vi "DARPA_DoubleJ_20220811_Arduino_ver.vi"() -> ()   [LabVIEW 2021]
uses:
  <vilib>/Instr/_visa.llb/VISA Configure Serial Port (Instr).vi
  <vilib>/FPGAPlugInAG/PCIe-7857/niLvFpga_Open_PCIe-7857.vi
  <vilib>/rvi/interface/common/dynamic/niFpgaDynamicAddResources.vi
  <vilib>/Utility/error.llb/Error Cluster From Error Code.vi
  <vilib>/rvi/errors/niLvFpgaAdjustHostInterfaceError.vi
  <vilib>/FPGAPlugInAG/Dynamic/niLvFpga_Close_Dynamic.vi
  <vilib>/rvi/interface/nirviOpenFPGA/nirviOpenFPGA.xnode
  FPGA Bitfiles/darpatransitionj_FPGATarget_DARPAFPGADoubleJ_E+A750Kw4Ow.lvbitx
  DARPA_FPGA_DoubleJ_20220715.vi
  <vilib>/rvi/interface/nirviReadWriteControl/nirviReadWriteControl.xnode
  <vilib>/rvi/interface/nirviCloseFPGA/nirviCloseFPGA.xnode
  NiFpgaLv.dll
  <vilib>/rvi/interface/Simulation/niFpgaSimulationCallBeginRW.vi
panel:
  out "error out":errorcluster
  in  "stop":bool
  out "Image":u16[][](graph)
  in  "Display":bool=TRUE
  out "Total Frames":i32
  out "Elapsed Time":u32
  out "Software FPS":dbl
  out "Camera FPS":dbl
  in  "H Offset":i32 min=0 max=1604 step=4
  in  "H Width":i32 min=4 max=2304 step=4
  out "SMD":dbl
  out "SHO":i32
  in  "V Offset":i32 min=0 max=1604 step=4
  in  "V Width":i32 min=4 max=2304 step=4
  in  "Binning":u16(ring)=1 items=["1x1"=1, "2x2"=2, "4x4"=4]
  out "SHW":i32
  out "SVO":i32
  out "SVW":i32
  in  "Scan Mode":dbl min=1.0 max=3.0 step=1.0
  in  "Exposure":dbl min=6.576470588235294e-05 max=10.000017235294118 step=1e-08
  out "EXP":dbl
  out "Camera Model":string
  out "Camera Version":string
  out "Camera Serial":string
  in  "Merger on":bool
  in  "ratiocontrol":dbl=1.0
  in  "Arduino COM port":refnum<visa-resource-name>="COM10"
  in  "Arduino \nshut down":bool=TRUE
  in  "Initializer":bool
  out "Serial debugger":string
  in  "PMT2 senstivity":bool
  in  "PMT1 senstivity":bool
  in  "Func amp":bool
  in  "Func Freq":bool
  in  "Func On time":bool
  in  "Func Delay":bool
  in  "PMT1 senstivity input":dbl=0.7 caption="0.5-0.75 V"
  in  "PMT2 senstivity input":dbl caption="0.5-0.75 V"
  in  "Func amp input":dbl=5.0 caption="0 - 5 V"
  in  "Func freq input":dbl=10000.0 caption="100 - 10k Hz"
  in  "Func on Time input":dbl=0.04 caption="0.01 - 1 s"
  in  "Func delay input":dbl caption="0.01 - 1 s"
  out "PMT2 sum":u64(graph)
  out "PMT1 sum":u64(graph)
  out "Unfiltered Signal 1":i16(graph)=643
  out "Filtered Signal 2":i16(graph)=-141
  out "Unfiltered Signal 2":i16(graph)=-138
  in  "Threshold1":dbl=9000.0
  in  "Threshold2":dbl
  out "LabView Timer (sec)":dbl
  out "sample diff":u64
  out "t1 (sample)":u64
  out "t0 (sample)":u64
  out "PMT1 sum":u64
  out "PMT2 sum":u64
  out "Droplet lock on":bool
  out "Filtered Signal1":dbl=373.0
  out "Filtered Signal2":dbl=-141.0
  out "Droplet counter":u64
  out "Unfiltered Signal1":dbl=643.0
  out "Unfiltered Signal2":dbl=-138.0
  in  "Droplet width [ms]":dbl
  in  "determine ratio (xx.xx)":dbl
  out "FPGA loop counter":u64=4737476
  out "Sorted droplet counter":u64
  out "Sort":bool
  in  "FPGA initializer":bool=TRUE
  out "FPGA timer (sec)":dbl=4.737476
  out "FPGA freq":dbl=1000000.0
  out "LabView freq":dbl=8547.008547008547
  out "Filtered Signal 1":i16(graph)=373
  out "PMT1/PMT2":dbl
  out "PMT1/PMT2 (graph)":dbl(graph)
  in  "Shut down program":bool=TRUE
  in  "Set rate1":dbl=1000.0 format="%#_4g"
  in  "Units1":string(combo)="uh"
  in  "Target Vol1":dbl=1000.0 caption="Target Vol (ul)"
  in  "Direction1":string(combo)="inf"
  in  "Send1":bool
  out "Max rate1":dbl=53066.71422466229 format="%#_4g"
  out "Min rate1":dbl=0.7293489203037584 caption="Min rate" format="%#_4g"
  in  "Pump1\nStart/Stop":bool
  out "Dispensed1":string
  in  "Reset1":bool
  out "Remains1":string="1.000000ML"
  in  "Syringe Selection1":string(combo)="BDP1MM"
  in  "dia1 (mm)":dbl=0.1 caption="Set Diameter (mm)" min=0.1 max=50.0
  out "Diameter1 (mm)":dbl=4.699
  in  "Set rate2":dbl=1500.0 format="%#_4g"
  in  "Units2":string(combo)="uh"
  in  "Target Vol2":dbl=2000.0 caption="Target Vol (ul)"
  in  "Direction2":string(combo)="inf"
  out "Max rate2":dbl=54911.979673505 format="%#_4g"
  out "Min rate2":dbl=0.7547102486326527 caption="Min rate" format="%#_4g"
  in  "Syringe Selection2":string(combo)="BDP1MM"
  in  "dia2 (mm)":dbl=0.1 caption="Set Diameter (mm)" min=0.1 max=50.0
  out "Diameter2 (mm)":dbl=4.78
  in  "Set rate3":dbl=1000.0 format="%#_4g"
  in  "Units3":string(combo)="uh"
  in  "Target Vol3":dbl=2000.0 caption="Target Vol (ul)"
  in  "Direction3":string(combo)="inf"
  out "Max rate3":dbl=54911.979673505 format="%#_4g"
  out "Min rate3":dbl=0.7547102486326527 caption="Min rate" format="%#_4g"
  in  "Syringe Selection3":string(combo)="BDP1MM"
  in  "dia3 (mm)":dbl=0.1 caption="Set Diameter (mm)" min=0.1 max=50.0
  out "Diameter3 (mm)":dbl=4.78
  in  "Pump2\nStart/Stop":bool
  in  "Pump3\nStart/Stop":bool
  out "Dispensed2":string
  out "Dispensed3":string
  out "Remains2":string="2.000000ML"
  out "Remains3":string="2.000000ML"
  in  "Reset2":bool
  in  "Reset3":bool
  in  "Reset4":bool
  in  "Syringe COM port":refnum<visa-resource-name>="COM11"
  out "Baud Rate":string="19200"
  in  "Output file path":string="D:\\PhD\\00TAMU\\1.research\\nanoBioSystem\\1.projects\\1.DARPA_iSENTRY\\2.src\\LabView\\transition\\FPGA7857_2020\\output files"
  in  "file name":string="tmep"
  out "Confirm path":string="C:\\Data_JJH\\1.Research\\1.projects\\1.DARPA_iSENTRY\\2.src\\LabView\\transition\\FPGA7857_2020\\output files\\20220811 sorting empty 1to500 1.xls"
  out "Data File Ptr":refnum<file>
  # "For inner peace of developers"
  # "Communication Setting"
  # "Sorting Status"
  # "[Pump1] Syringe Setting"
  # "Arduino setting"
  # "[Pump2] Syringe Setting"
  # "PMT display"
  # "Cockpit"
  # "[Pump3] Syringe Setting"
  # "File saving option"
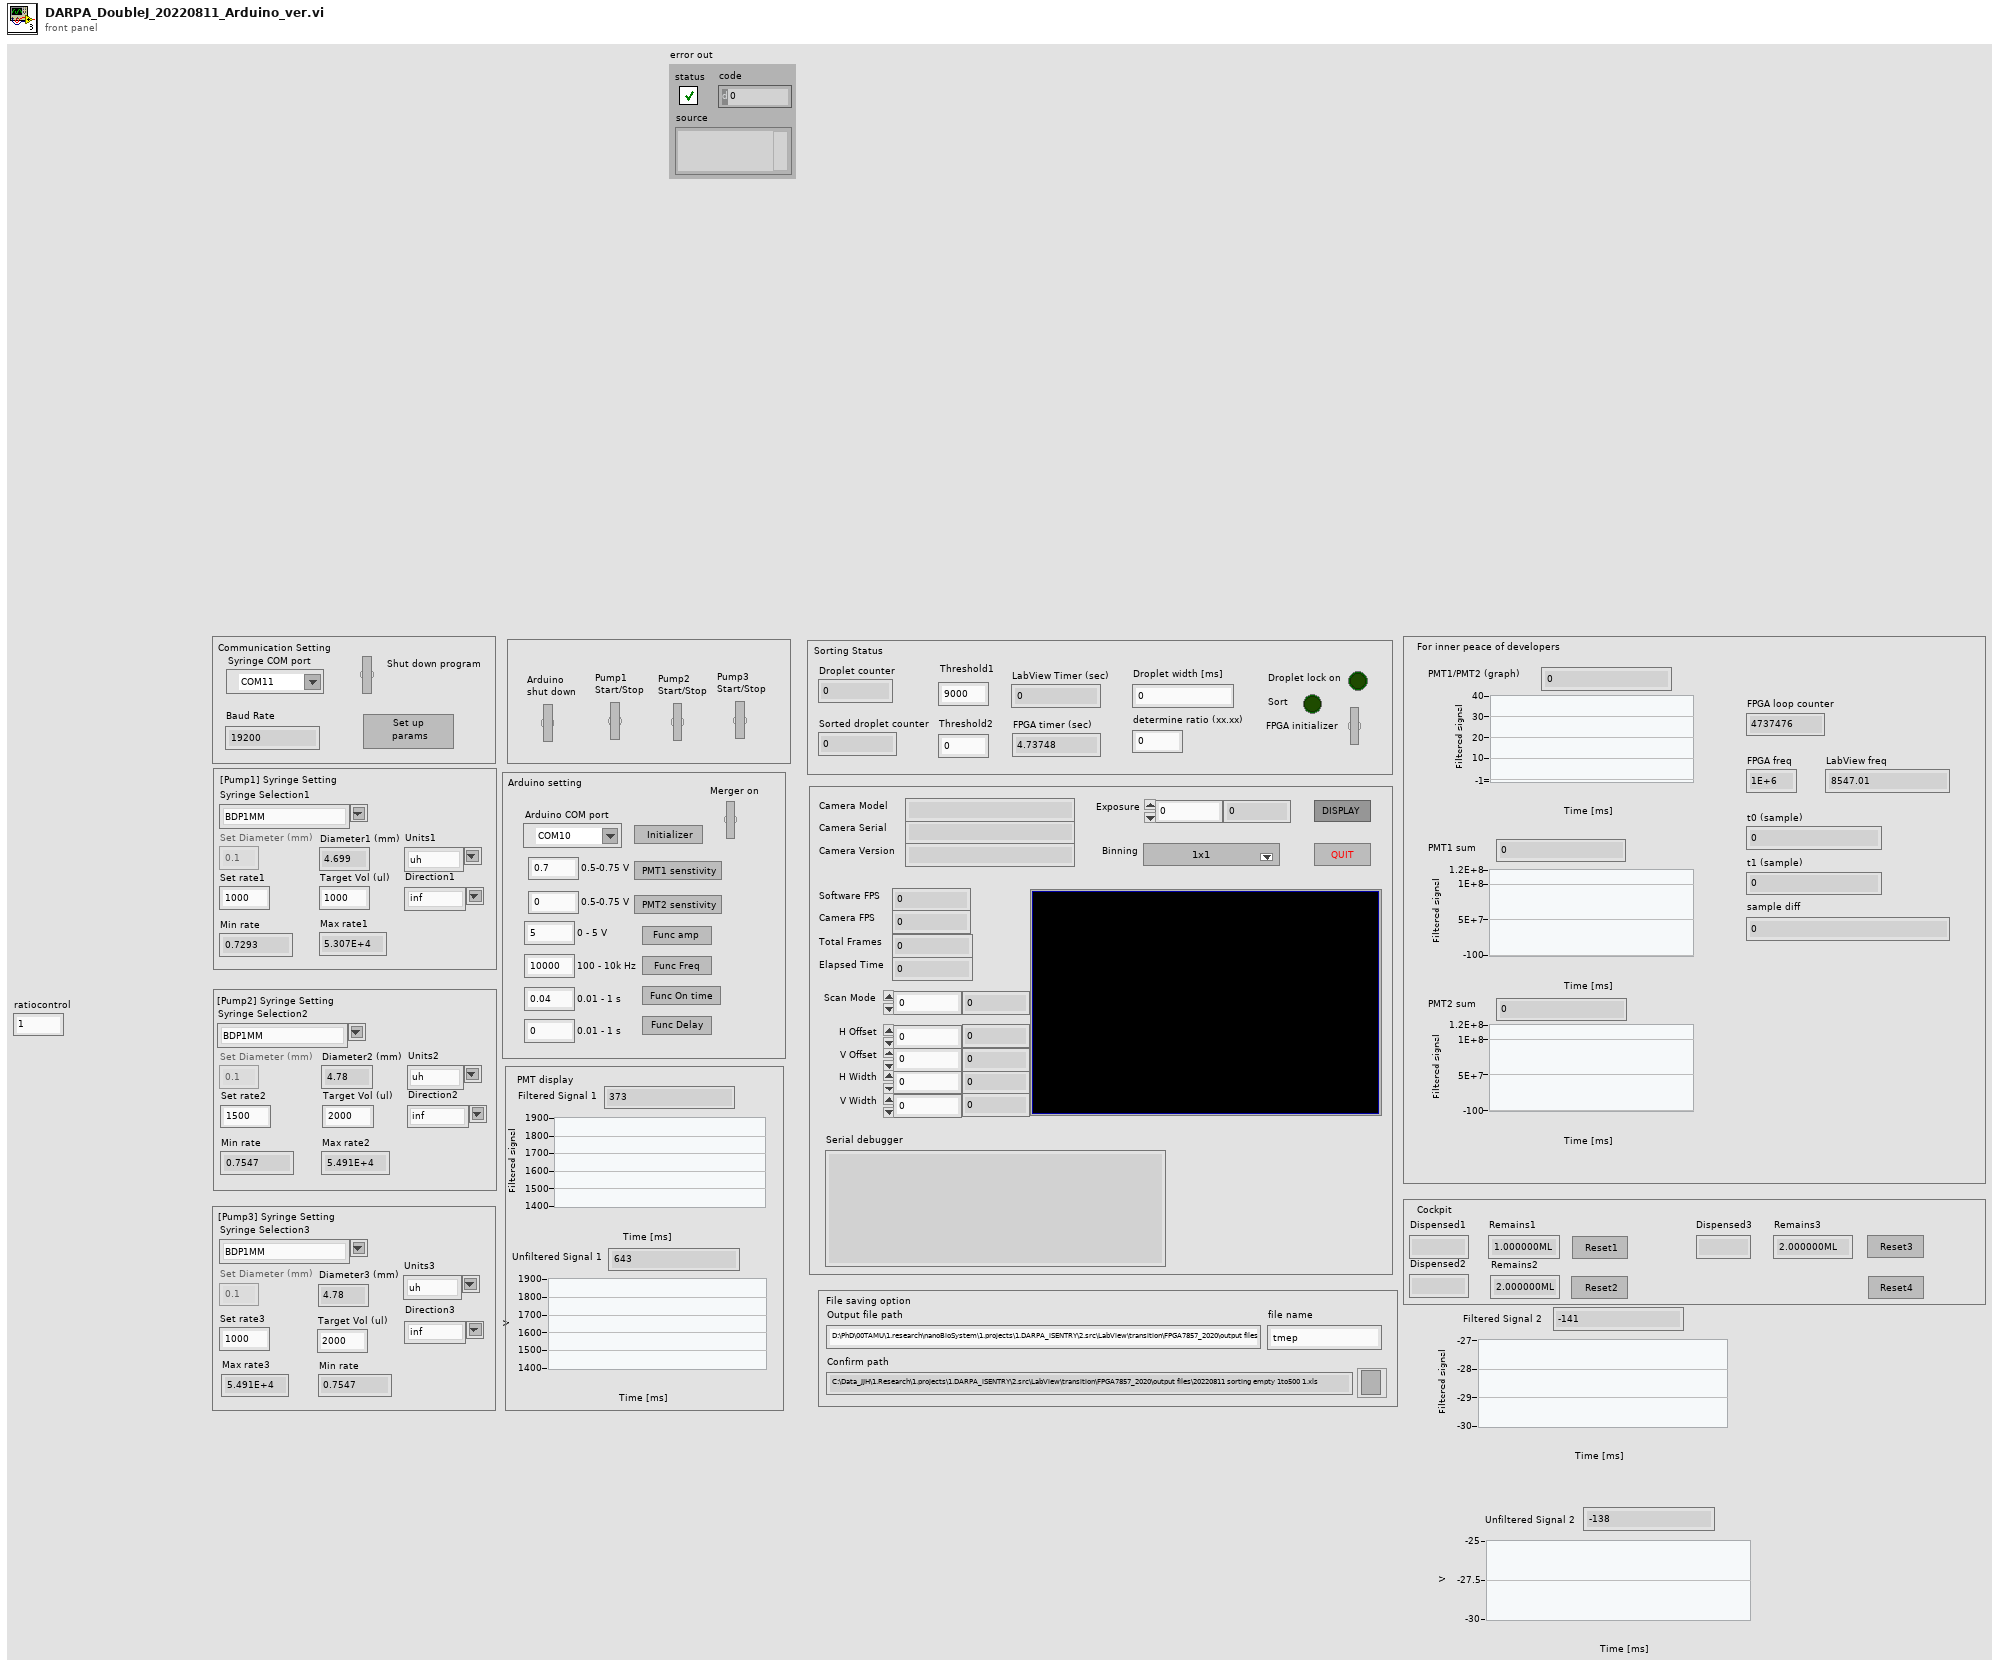
[diagram p1: front panel]
types:
  T1 = enum16{"open", "replace", "create", "open or create", "replace or create", "replace or create with confirmation"}
  T2 = enum8{"Enabled", "Disabled", "Disabled and Grayed Out"}
  T3 = cluster{"Model":string, "Camera ID":string, "Firmware":string}
  T4 = typedef "LVMinMaxIncTypeDef.ctl" = cluster{"Minimum":dbl, "Maximum":dbl, "Increment":dbl}
  T5 = cluster{"H Offset":cluster{"Value":i32, "Limits":T4}, "V Offset":cluster{"Value":i32, "Limits":T4}, "H Size":cluster{"Value":i32, "Limits":T4}, "V Size":cluster{"Value":i32, "Limits":T4}}
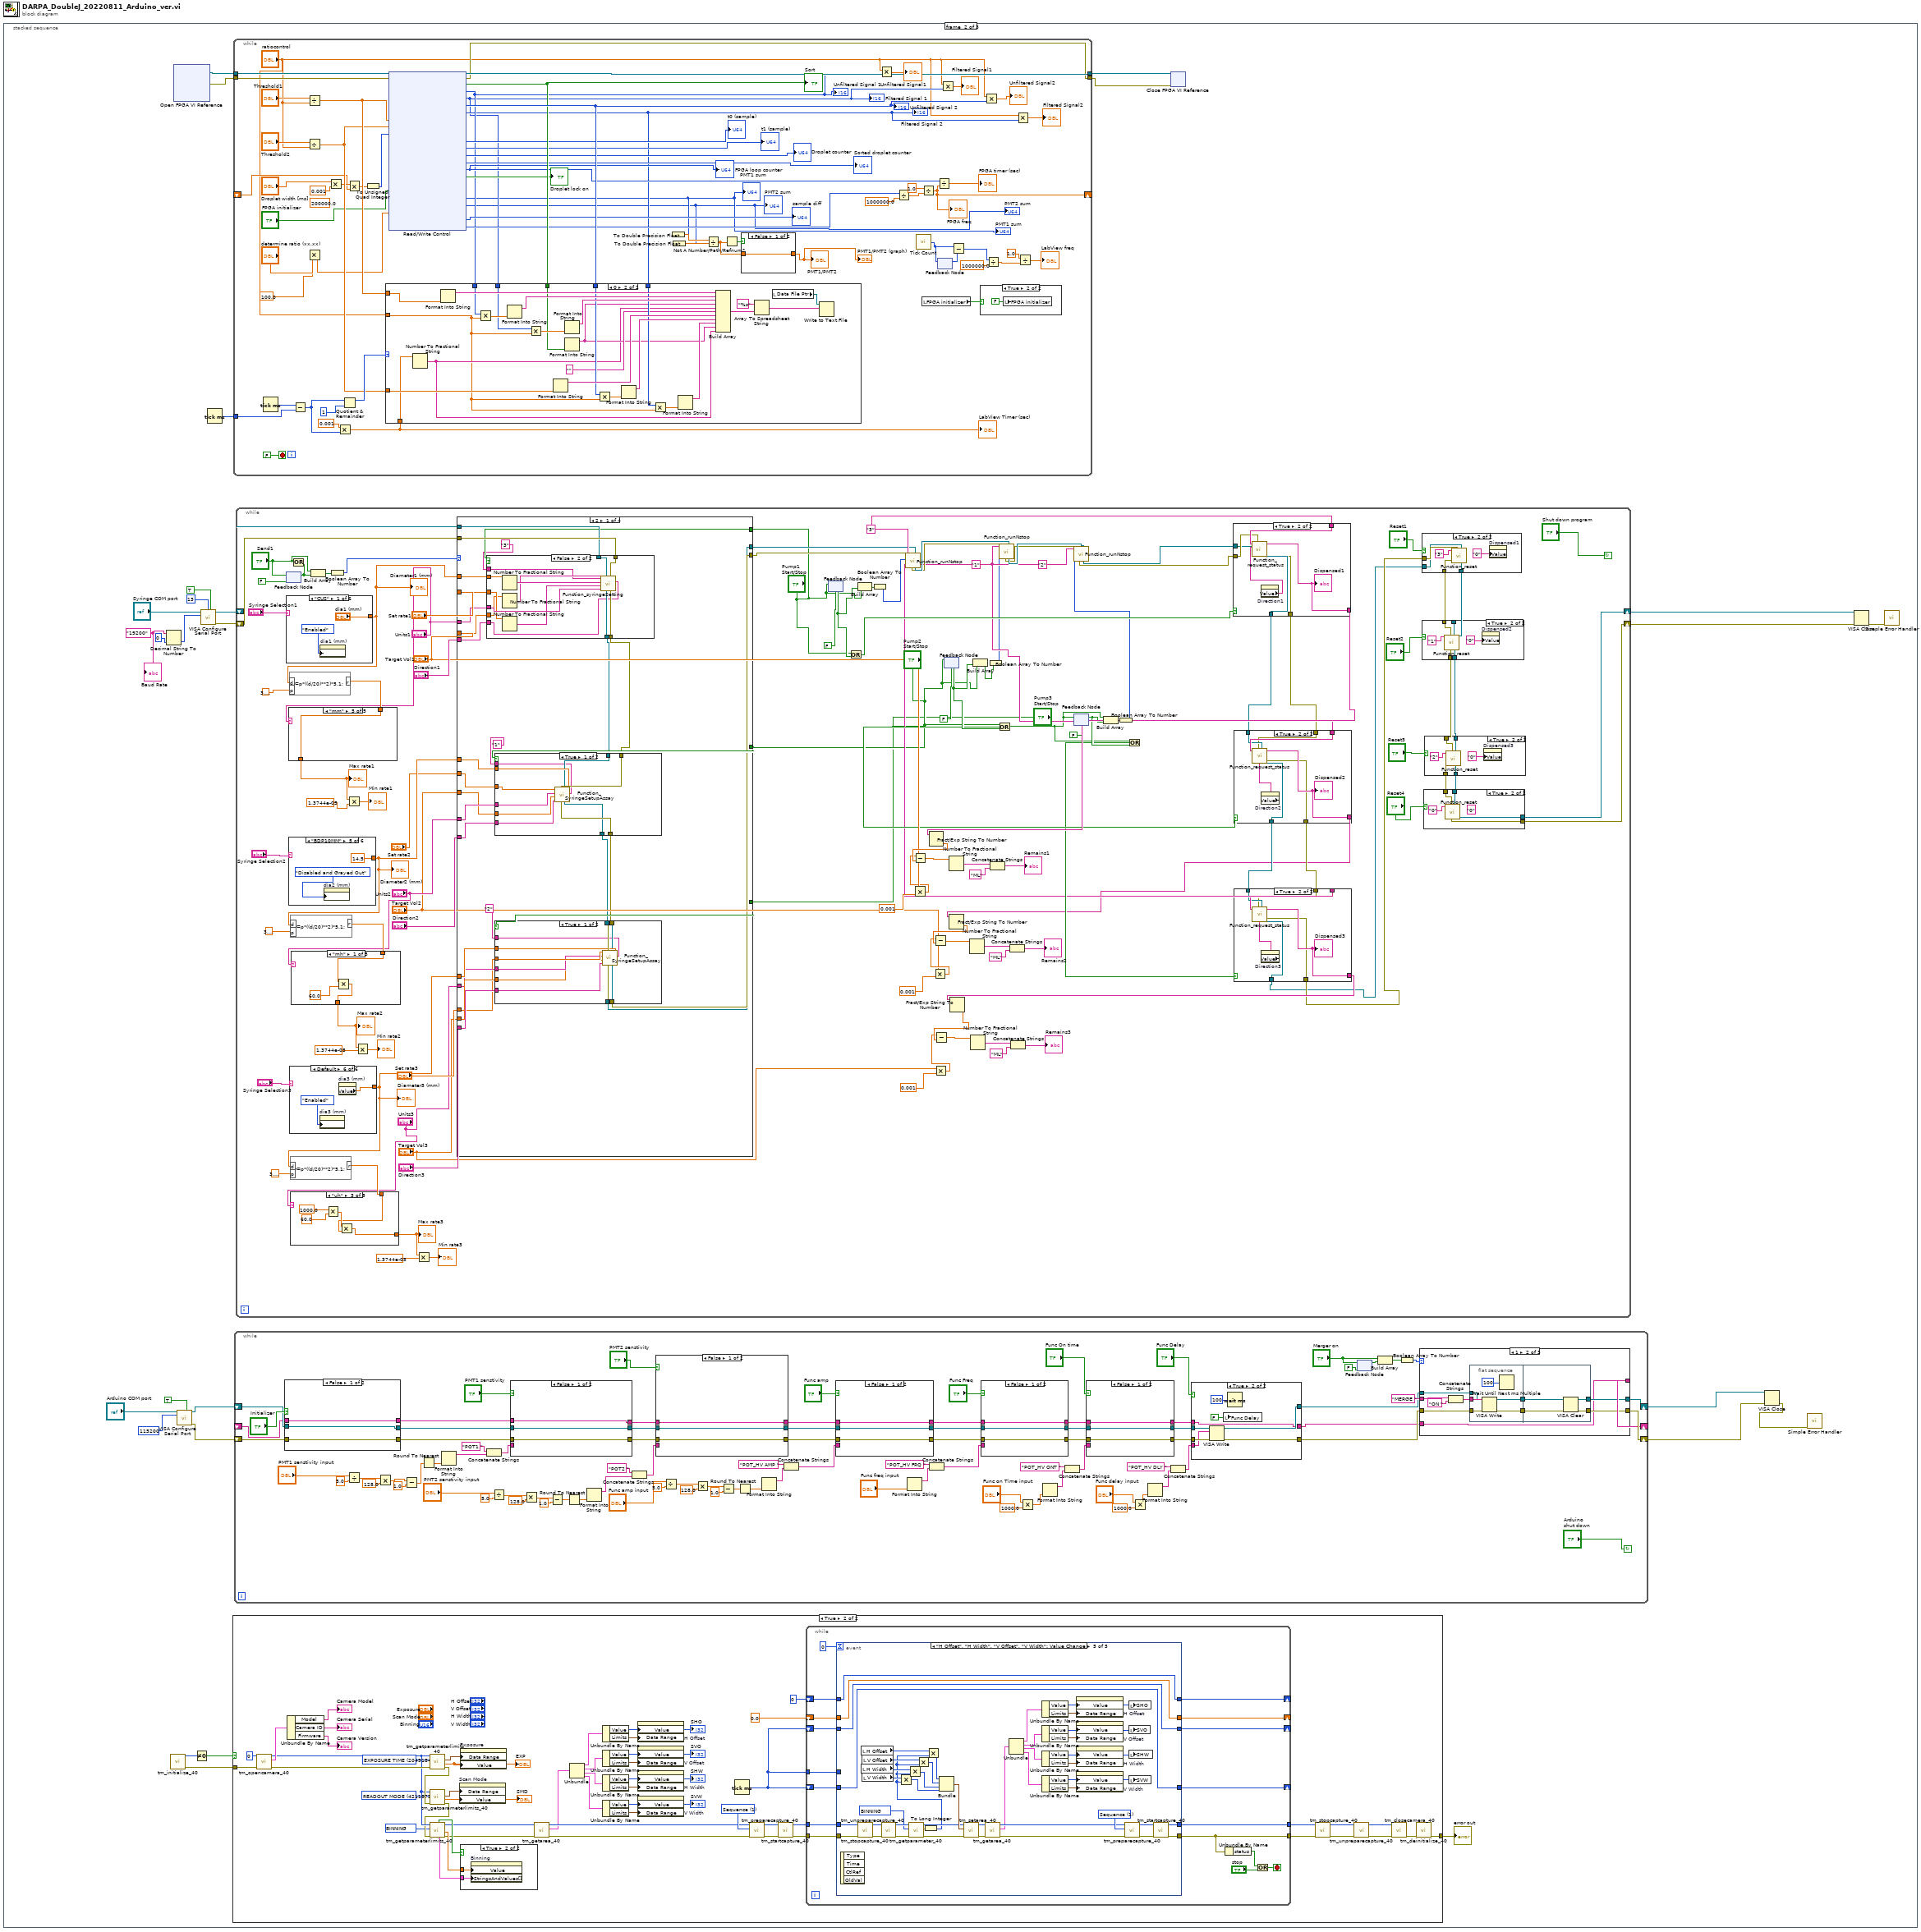
[diagram p0: block diagram]
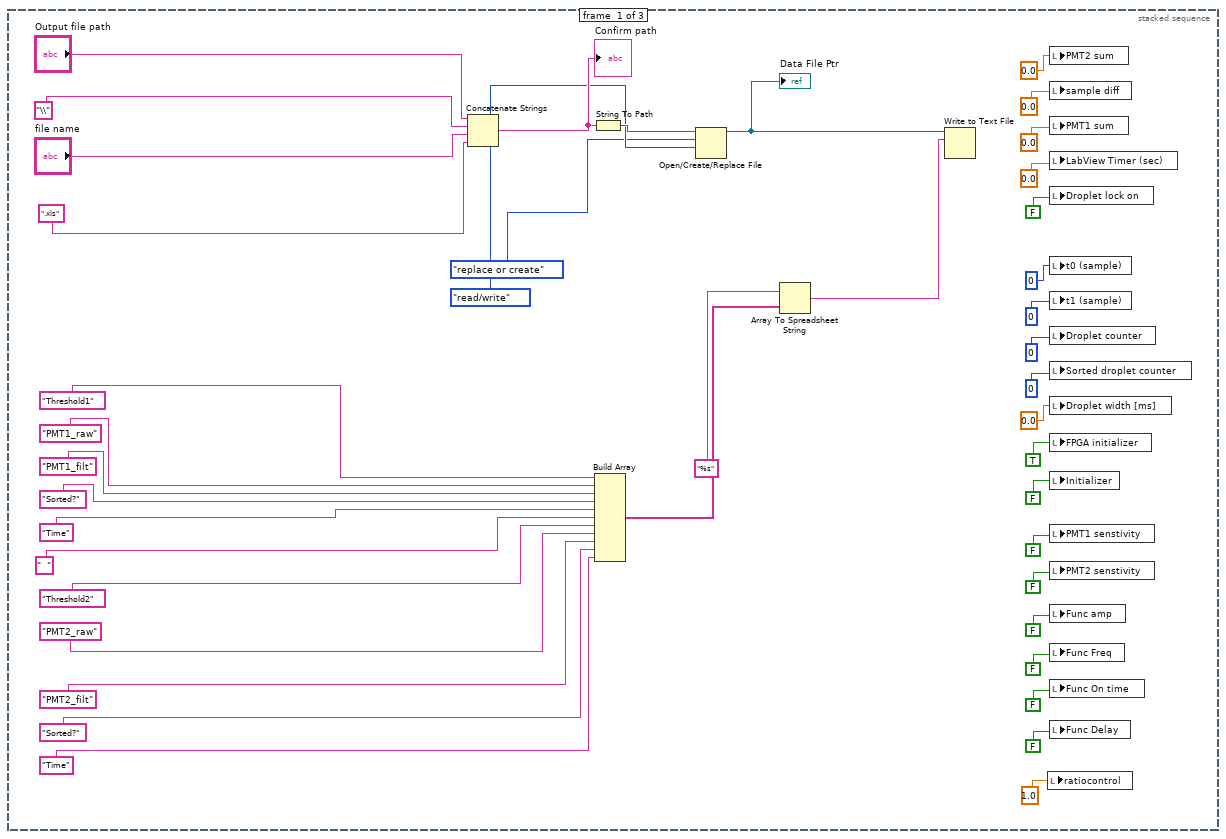
[diagram p2: hidden frame]
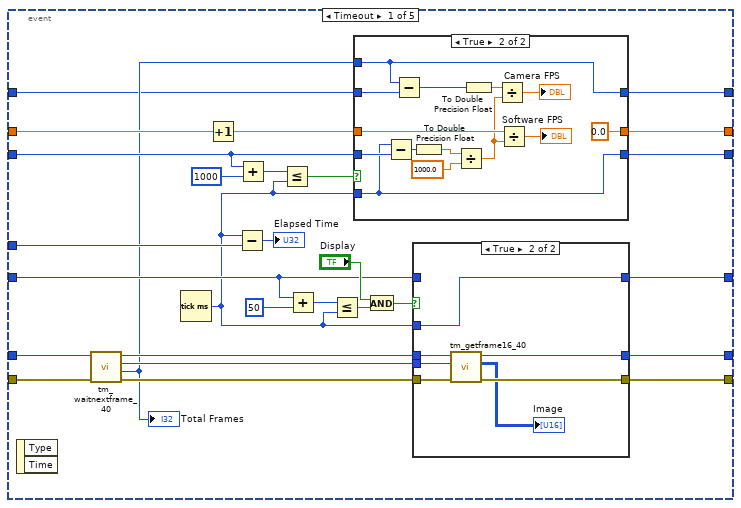
[diagram p5: hidden frame]
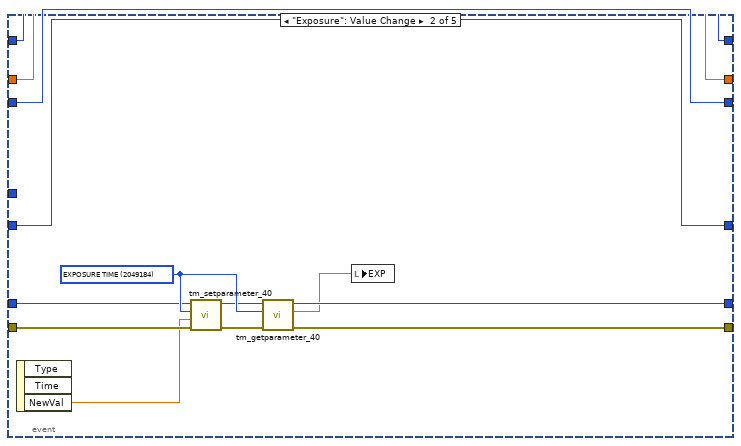
[diagram p8: hidden frame]
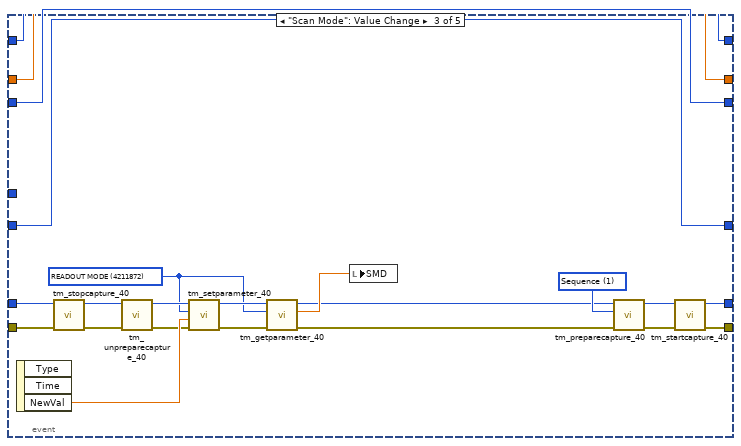
[diagram p9: hidden frame]
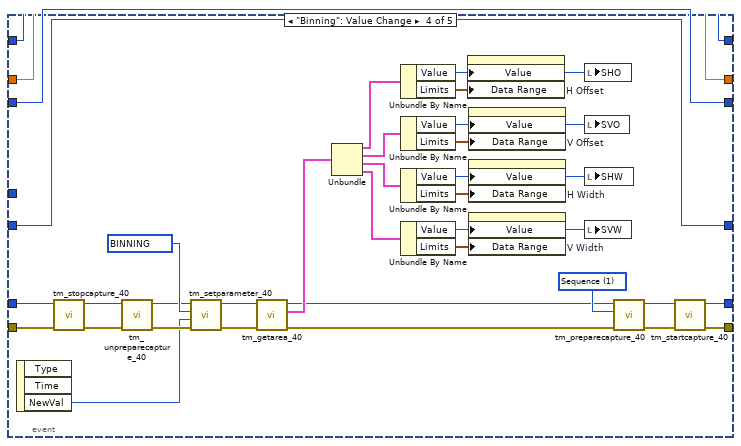
[diagram p10: hidden frame]
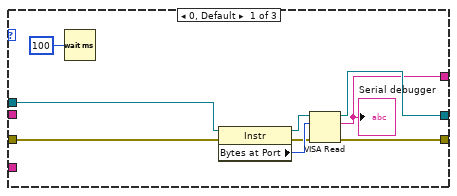
[diagram p11: hidden frame]
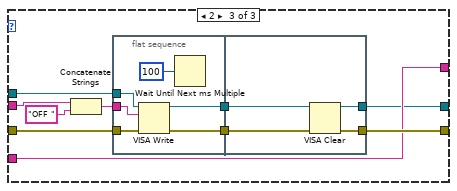
[diagram p12: hidden frame]
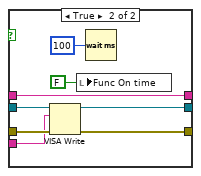
[diagram p14: hidden frame]
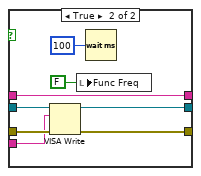
[diagram p15: hidden frame]
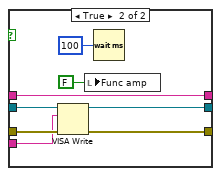
[diagram p16: hidden frame]
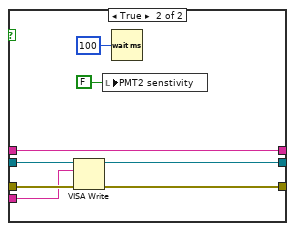
[diagram p17: hidden frame]
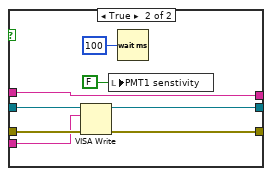
[diagram p18: hidden frame]
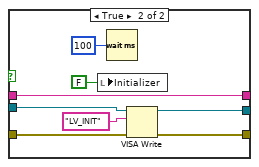
[diagram p19: hidden frame]
diagram:
  n1 = stacked-sequence {
    frame #0 {
      n2 = Concatenate Strings("Output file path", "\\" ("string"), "file name", ".xls" ("string")) -> (w41:string)
      "Confirm path" <- w41
      n3 = String To Path(string=w41) -> (path=w42:path)
      n4 = Build Array("Threshold1", "PMT1_raw", "PMT1_filt", "Sorted?", "Time", "  ", "Threshold2", "PMT2_raw", "PMT2_filt", "Sorted?", "Time") -> (w34:string[])
      n5 = Open/Create/Replace File(file path (use dialog)=w42, operation (0:open)=T1."replace or create", access (0:read/write)=enum16{"read/write", "read-only", "write-only"}."read/write") -> (refnum out=w20:refnum<file>)  [unwired: 3 in, 2 out]
      "Data File Ptr" <- w20
      n6 = Array To Spreadsheet String(array=w34, 3:"%s") -> (spreadsheet string=w22:string)  [unwired: 1 in]
      n7 = Write to Text File(file (use dialog)=w20, text=w22) -> ()  [unwired: 2 in, 3 out]
      n8 = local write "ratiocontrol"(1.0 ("ratiocontrol")) -> ()
      n9 = local write "PMT2 sum"(0.0 ("now")) -> ()
      n10 = local write "sample diff"(0.0 ("sample diff")) -> ()
      n11 = local write "PMT1 sum"(0.0 ("PMT1 sum")) -> ()
      n12 = local write "LabView Timer (sec)"(0.0 ("PMT2 sum")) -> ()
      n13 = local write "Droplet lock on"(FALSE ("Droplet lock on")) -> ()
      n14 = local write "t0 (sample)"(u64 0 ("t0 (sample)")) -> ()
      n15 = local write "t1 (sample)"(u64 0 ("t1 (sample)")) -> ()
      n16 = local write "Droplet counter"(u64 0 ("Droplet counter")) -> ()
      n17 = local write "Sorted droplet counter"(u64 0 ("Sorted droplet counter")) -> ()
      n18 = local write "Droplet width [ms]"(0.0 ("Time compensation [ms]")) -> ()
      n19 = local write "FPGA initializer"(TRUE ("FPGA initializer")) -> ()
      n20 = local write "Initializer"(FALSE ("FPGA initializer")) -> ()
      n21 = local write "PMT1 senstivity"(FALSE ("FPGA initializer")) -> ()
      n22 = local write "PMT2 senstivity"(FALSE ("FPGA initializer")) -> ()
      n23 = local write "Func amp"(FALSE ("FPGA initializer")) -> ()
      n24 = local write "Func Freq"(FALSE ("FPGA initializer")) -> ()
      n25 = local write "Func On time"(FALSE ("FPGA initializer")) -> ()
      n26 = local write "Func Delay"(FALSE ("FPGA initializer")) -> ()
    }
    frame #1 {
      w60 = "19200" ("Baud Rate")
      n27 = Decimal String To Number(string=w60, default (0L)=u32 0 ("default (0 I32)")) -> (number=w63:u32)  [unwired: 1 in, 1 out]
      n28 = call <userlib>:"tm_initialize_40.vi"() -> ("error out"=w44:errorcluster, "Number Of Cameras"=w43:u32)  [unwired: 8 in, 2 out]
      n29 = xnode "Open FPGA VI Reference"() -> ("FPGA VI Reference Out"=w70:refnum<k20>, "error out"=w69:errorcluster)  [unwired: 2 in]
      n30 = call-poly "VISA Configure Serial Port"("VISA resource name"="Arduino COM port", "Enable Termination\nChar (T)"=TRUE ("Enable Termination\nChar (T)"), "baud rate (9600)"=u32 115200) -> ("VISA resource name out"=w50:refnum<visa-resource-name>, "error out"=w49:errorcluster)  [unwired: 11 in]
      n31 = Not Equal To 0?(x=w43) -> (x != 0?=w46:bool)
      n32 = call-poly "VISA Configure Serial Port"("VISA resource name"="Syringe COM port", "termination char\n(0xA = '\\n' = LF)"=u8 13 ("termination char\n(0xA = '\\n' = LF)"), "Enable Termination\nChar (T)"=TRUE ("Enable Termination\nChar (T)"), "baud rate (9600)"=w63) -> ("VISA resource name out"=w59:refnum<visa-resource-name>, "error out"=w58:errorcluster)  [unwired: 10 in]
      n33 = Tick Count (ms)() -> (millisecond timer value=w66:u32)
      n34 = case shown="True" w46 {
        tunnel: [w71 w121] -> w45
        tunnel: w44 -> [w71 w124]
        frame False {
        }
        frame True {
          w93 = u32 2049184 items=["BINNING"=4215968, "BITS PER CHANNEL"=4342976, "ACTIVE VIEW INDEX"=4343136, "CCD MODE"=4212384, "SENSOR MODE"=4212128, "READOUT MODE"=4211872, "EXPOSURE TIME"=2049184, "CONTRAST GAIN"=3163312, "CONTRAST OFFSET"=3163328, "LIGHT MODE"=2114720, "SENSITIVITY"=2114992, "WHITE BALANCE"=3163568, "PHOTON IMAGING MODE"=2115200, "HIGH DYNAMIC RANGE MODE"=3163360, "TRIGGER SOURCE"=1066144, "TRIGGER ACTIVE"=1066160, "TRIGGER MODE"=1066400, "TRIGGER POLARITY"=1066416, "TRIGGER GLOBAL EXPOSURE"=2049680, "FIRST TRIGGER BEHAVIOR"=2049696, "TRIGGER TIMES"=1066448, "OUTPUT TRIGGER POLARITY"=1852592, "OUTPUT TRIGGER DELAY"=1852624, "OUTPUT TRIGGER PERIOD"=1852640, "TEMPERATURE"=2115232, "TEMPERATURE TARGET"=2115264, "SENSOR COOLER FAN"=2115296, "MECHANICAL SHUTTER"=2115488, "BACK FOCUS POSITION"=8422304, "FRAMEBUNDLE MODE"=4346784, "FRAMEBUNDLE NUMBER"=4346800, "LINEBUNDLE HEIGHT"=4212192, "TRIGGER CONNECTOR"=1066432, "IMAGE PIXEL TYPE"=4343296, "OUTPUT TRIGGER KIND"=1852656, "READOUT DIRECTION"=4211904, "CHANNEL SYNC"=1852352] ("Parameter")
          w94 = u32 4211872 items=["BINNING"=4215968, "BITS PER CHANNEL"=4342976, "ACTIVE VIEW INDEX"=4343136, "CCD MODE"=4212384, "SENSOR MODE"=4212128, "READOUT MODE"=4211872, "EXPOSURE TIME"=2049184, "CONTRAST GAIN"=3163312, "CONTRAST OFFSET"=3163328, "LIGHT MODE"=2114720, "SENSITIVITY"=2114992, "WHITE BALANCE"=3163568, "PHOTON IMAGING MODE"=2115200, "HIGH DYNAMIC RANGE MODE"=3163360, "TRIGGER SOURCE"=1066144, "TRIGGER ACTIVE"=1066160, "TRIGGER MODE"=1066400, "TRIGGER POLARITY"=1066416, "TRIGGER GLOBAL EXPOSURE"=2049680, "FIRST TRIGGER BEHAVIOR"=2049696, "TRIGGER TIMES"=1066448, "OUTPUT TRIGGER POLARITY"=1852592, "OUTPUT TRIGGER DELAY"=1852624, "OUTPUT TRIGGER PERIOD"=1852640, "TEMPERATURE"=2115232, "TEMPERATURE TARGET"=2115264, "SENSOR COOLER FAN"=2115296, "MECHANICAL SHUTTER"=2115488, "BACK FOCUS POSITION"=8422304, "FRAMEBUNDLE MODE"=4346784, "FRAMEBUNDLE NUMBER"=4346800, "LINEBUNDLE HEIGHT"=4212192, "TRIGGER CONNECTOR"=1066432, "IMAGE PIXEL TYPE"=4343296, "OUTPUT TRIGGER KIND"=1852656, "READOUT DIRECTION"=4211904, "CHANNEL SYNC"=1852352] ("Parameter")
          w95 = u32 4215968 items=["BINNING"=4215968, "BITS PER CHANNEL"=4342976, "ACTIVE VIEW INDEX"=4343136, "CCD MODE"=4212384, "SENSOR MODE"=4212128, "READOUT MODE"=4211872, "EXPOSURE TIME"=2049184, "CONTRAST GAIN"=3163312, "CONTRAST OFFSET"=3163328, "LIGHT MODE"=2114720, "SENSITIVITY"=2114992, "WHITE BALANCE"=3163568, "PHOTON IMAGING MODE"=2115200, "HIGH DYNAMIC RANGE MODE"=3163360, "TRIGGER SOURCE"=1066144, "TRIGGER ACTIVE"=1066160, "TRIGGER MODE"=1066400, "TRIGGER POLARITY"=1066416, "TRIGGER GLOBAL EXPOSURE"=2049680, "FIRST TRIGGER BEHAVIOR"=2049696, "TRIGGER TIMES"=1066448, "OUTPUT TRIGGER POLARITY"=1852592, "OUTPUT TRIGGER DELAY"=1852624, "OUTPUT TRIGGER PERIOD"=1852640, "TEMPERATURE"=2115232, "TEMPERATURE TARGET"=2115264, "SENSOR COOLER FAN"=2115296, "MECHANICAL SHUTTER"=2115488, "BACK FOCUS POSITION"=8422304, "FRAMEBUNDLE MODE"=4346784, "FRAMEBUNDLE NUMBER"=4346800, "LINEBUNDLE HEIGHT"=4212192, "TRIGGER CONNECTOR"=1066432, "IMAGE PIXEL TYPE"=4343296, "OUTPUT TRIGGER KIND"=1852656, "READOUT DIRECTION"=4211904, "CHANNEL SYNC"=1852352] ("Parameter")
          w119 = 1 items=["Snap", "Sequence"] ("Capture mode")
          n35 = call <userlib>:"tm_opencamera_40.vi"("error in (no error)"=w124, "Camera Index"=u32 0) -> ("error out"=w102:errorcluster, "Camera Details"=w106:T3, "Handle out"=w100:u32)  [unwired: 7 in]
          n36 = Unbundle By Name(w106) -> ("Model"=→"Camera Model":string, "Camera ID"=→"Camera Serial":string, "Firmware"=→"Camera Version":string)
          n37 = call <userlib>:"tm_getparameterlimits_40.vi"("error in (no error)"=w102, "Parameter"=w93, "Handle in"=w100) -> ("error out"=w101:errorcluster, "default"=w85:dbl, "Range"=w86:cluster{"min":dbl, "max":dbl, "step":dbl})  [unwired: 2 in, 4 out]
          "EXP" <- w85
          n38 = call <userlib>:"tm_getparameterlimits_40.vi"("error in (no error)"=w101, "Parameter"=w94, "Handle in"=w100) -> ("error out"=w99:errorcluster, "default"=w87:dbl, "Range"=w88:cluster{"min":dbl, "max":dbl, "step":dbl})  [unwired: 2 in, 4 out]
          "SMD" <- w87
          n39 = call <userlib>:"tm_getparameterlimits_40.vi"("error in (no error)"=w99, "Parameter"=w95, "Handle in"=w100) -> ("error out"=w92:errorcluster, "default"=w97:dbl, "Handle out"=w91:u32, "Value Names"=w96:cluster{"Name":string, "Value":dbl}[], "Writable"=w98:bool)  [unwired: 2 in, 2 out]
          n40 = property on="Scan Mode" class="DigNum (strict)"("Data Range"=w88, "Value"=w87) -> ()  [unwired: 2 in, 2 out]
          n41 = property on="Exposure" class="DigNum (strict)"("Data Range"=w86, "Value"=w85) -> ()  [unwired: 2 in, 2 out]
          n42 = case shown="True" w98 {
            tunnel: w96 -> [_ w126]
            tunnel: w97 -> [_ w125]
            frame False {
            }
            frame True {
              n43 = property on="Binning" class="Ring (strict)"("Value"=w125, "StringsAndValues[]"=w126) -> ()  [unwired: 2 in, 2 out]
            }
          }
          n44 = call <userlib>:"tm_getarea_40.vi"("error in (no error)"=w92, "Handle in"=w91) -> ("error out"=w90:errorcluster, "Sub Region"=w80:T5, "Handle out"=w89:u32)  [unwired: 7 in]
          n45 = Unbundle(w80) -> ("H Offset"=w84:cluster{"Value":i32, "Limits":T4}, "V Offset"=w83:cluster{"Value":i32, "Limits":T4}, "H Size"=w82:cluster{"Value":i32, "Limits":T4}, "V Size"=w81:cluster{"Value":i32, "Limits":T4})
          n46 = Unbundle By Name(w84) -> ("Value"=w79:i32, "Limits"=w78:T4)
          "SHO" <- w79
          n47 = Unbundle By Name(w83) -> ("Value"=w73:i32, "Limits"=w72:T4)
          "SVO" <- w73
          n48 = Unbundle By Name(w82) -> ("Value"=w75:i32, "Limits"=w74:T4)
          "SHW" <- w75
          n49 = Unbundle By Name(w81) -> ("Value"=w77:i32, "Limits"=w76:T4)
          "SVW" <- w77
          n50 = property on="H Offset" class="DigNum (strict)"("Value"=w79, "Data Range"=w78) -> ()  [unwired: 2 in, 2 out]
          n51 = property on="V Offset" class="DigNum (strict)"("Value"=w73, "Data Range"=w72) -> ()  [unwired: 2 in, 2 out]
          n52 = property on="H Width" class="DigNum (strict)"("Value"=w75, "Data Range"=w74) -> ()  [unwired: 2 in, 2 out]
          n53 = property on="V Width" class="DigNum (strict)"("Value"=w77, "Data Range"=w76) -> ()  [unwired: 2 in, 2 out]
          n54 = Tick Count (ms)() -> (millisecond timer value=w114:u32)
          n55 = call <userlib>:"tm_preparecapture_40.vi"("error in (no error)"=w90, "Capture mode"=w119, "Handle in"=w89) -> ("error out"=w117:errorcluster, "Handle out"=w118:u32)  [unwired: 5 in, 2 out]
          n56 = call <userlib>:"tm_startcapture_40.vi"("error in (no error)"=w117, "Handle in"=w118) -> ("error out"=w116:errorcluster, "Handle out"=w115:u32)  [unwired: 8 in]
          n57 = while {
            tunnel: w116 -> [w133]
            tunnel: [w131] -> w113
            tunnel: [w130] -> w112
            shift-right: [w139] -> _
            shift-left: w114 -> [w137]
            shift-right: [w140] -> _
            shift-left: 0.0 -> [w138]
            shift-right: [w132] -> _
            shift-left: w114 -> [w135]
            tunnel: w115 -> [w134]
            tunnel: w114 -> [w136]
            shift-right: [w127] -> _
            shift-left: 0 -> [w128]
            stop <- w141 stop-if-true
            n58 = event shown="[4] \"H Offset\", \"H Width\", \"V Offset\", \"V Width\": Value Change" {
              selector: _ -> [_ _ _ _ _]
              dyn-events: _ -> [_ _ _ _ _]
              timeout: 0 -> [_ _ _ _ _]
              tunnel: [w148 w209 w231 w260 w306] -> w140
              tunnel: [w147 w210 w232 w261 w307] -> w139
              tunnel: w138 -> [w157 w209 w231 w260 w306]
              tunnel: w137 -> [w150 w210 w232 w261 w307]
              tunnel: w136 -> [w153 _ _ _ _]
              tunnel: w135 -> [w158 w211 w233 w267 w313]
              tunnel: w134 -> [w160 w204 w228 w259 w304]
              tunnel: w133 -> [w159 w206 w227 w258 w303]
              tunnel: [w156 w211 w233 w267 w313] -> w132
              tunnel: [w155 w201 w222 w262 w308] -> w131
              tunnel: [w154 w199 w223 w263 w309] -> w130
              tunnel: w128 -> [w145 w208 w221 w255 w300]
              tunnel: [w144 w208 w221 w255 w300] -> w127
              event Timeout {
                n59 = event-data() -> ()  [unwired: 1 in, 2 out]
                n60 = call <userlib>:"tm_waitnextframe_40.vi"("error in (no error)"=w159, "Handle in"=w160) -> ("error out"=w164:errorcluster, "Frame Count"=w146:i32, "Frame Index"=w163:i32, "Handle out"=w165:u32)  [unwired: 6 in]
                "Total Frames" <- w146
                n61 = Tick Count (ms)() -> (millisecond timer value=w152:u32)
                n62 = Increment(x=w157) -> (x+1=w149:dbl)
                n63 = Subtract(x=w152, y=w153) -> (x-y=→"Elapsed Time":u32)
                n64 = Add(x=w150, y=u32 1000) -> (x+y=w171:u32)
                n65 = Less Or Equal?(x=w171, y=w152) -> (x <= y?=w151:bool)
                n66 = Add(x=w158, y=u32 50) -> (x+y=w169:u32)
                n67 = Less Or Equal?(x=w169, y=w152) -> (x <= y?=w167:bool)
                n68 = case shown="True" w151 {
                  tunnel: w150 -> [w174 w183]
                  tunnel: [w174 w180] -> w147
                  tunnel: w149 -> [w173 w186]
                  tunnel: w152 -> [_ w180]
                  tunnel: [w173 0.0] -> w148
                  tunnel: w146 -> [_ w175]
                  tunnel: w145 -> [w172 w178]
                  tunnel: [w172 w175] -> w144
                  frame False {
                  }
                  frame True {
                    n69 = Subtract(x=w180, y=w183) -> (x-y=w182:u32)
                    n70 = Subtract(x=w175, y=w178) -> (x-y=w176:i32)
                    n71 = To Double Precision Float(number=w182) -> (double precision float=w188:dbl)
                    n72 = Divide(x=w188, y=1000.0) -> (x/y=w179:dbl)
                    n73 = To Double Precision Float(number=w176) -> (double precision float=w177:dbl)
                    n74 = Divide(x=w177, y=w179) -> (x/y=→"Camera FPS":dbl)
                    n75 = Divide(x=w186, y=w179) -> (x/y=→"Software FPS":dbl)
                  }
                }
                n76 = And(x="Display", y=w167) -> (x .and. y?=w162:bool)
                n77 = case shown="True" w162 {
                  tunnel: w158 -> [w191 _]
                  tunnel: w152 -> [_ w198]
                  tunnel: [w191 w198] -> w156
                  tunnel: w165 -> [w190 w197]
                  tunnel: w164 -> [w189 w196]
                  tunnel: [w190 w195] -> w155
                  tunnel: [w189 w194] -> w154
                  tunnel: w163 -> [_ w192]
                  frame False {
                  }
                  frame True {
                    n78 = call <userlib>:"tm_getframe16_40.vi"("error in (no error)"=w196, "Frame Index"=w192, "Handle in"=w197) -> ("error out"=w194:errorcluster, "Data"=→"Image":u16[][], "Handle out"=w195:u32)  [unwired: 5 in, 1 out]
                  }
                }
              }
              event "Exposure": Value Change {
                w207 = u32 2049184 items=["SENSOR MODE"=4212128, "CCD MODE"=4212384, "READOUT MODE"=4211872, "ACTIVE VIEW INDEX"=4343136, "BITS PER CHANNEL"=4342976, "IMAGE PIXEL TYPE"=4343296, "BINNING"=4215968, "EXPOSURE TIME"=2049184, "CONTRAST GAIN"=3163312, "CONTRAST OFFSET"=3163328, "LIGHT MODE"=2114720, "SENSITIVITY"=2114992, "PHOTON IMAGING MODE"=2115200, "HIGH DYNAMIC RANGE MODE"=3163360, "WHITE BALANCE"=3163568, "TEMPERATURE"=2115232, "TEMPERATURE TARGET"=2115264, "SENSOR COOLER FAN"=2115296, "LINEBUNDLE HEIGHT"=4212192, "MECHANICAL SHUTTER"=2115488, "BACK FOCUS POSITION"=8422304, "TRIGGER CONNECTOR"=1066432, "TRIGGER SOURCE"=1066144, "OUTPUT TRIGGER SOURCE"=1852576, "TRIGGER GLOBAL EXPOSURE"=2049680, "FIRST TRIGGER BEHAVIOR"=2049696, "CHANNEL SYNC"=1852352, "READOUT DIRECTION"=4211904, "PRE HSYNC COUNT"=1852704] ("Parameter")
                n79 = event-data() -> ("NewVal"=w205:dbl)  [unwired: 1 in, 2 out]
                n80 = call <userlib>:"tm_setparameter_40.vi"("error in (no error)"=w206, "Value in"=w205, "Parameter"=w207, "Handle in"=w204) -> ("error out"=w203:errorcluster, "Handle out"=w202:u32)  [unwired: 6 in]
                n81 = call <userlib>:"tm_getparameter_40.vi"("error in (no error)"=w203, "Parameter"=w207, "Handle in"=w202) -> ("error out"=w199:errorcluster, "Value out"=w200:dbl, "Handle out"=w201:u32)  [unwired: 6 in]
                n82 = local write "EXP"(w200) -> ()
              }
              event "Scan Mode": Value Change {
                w212 = u32 4211872 items=["SENSOR MODE"=4212128, "CCD MODE"=4212384, "READOUT MODE"=4211872, "ACTIVE VIEW INDEX"=4343136, "BITS PER CHANNEL"=4342976, "IMAGE PIXEL TYPE"=4343296, "BINNING"=4215968, "EXPOSURE TIME"=2049184, "CONTRAST GAIN"=3163312, "CONTRAST OFFSET"=3163328, "LIGHT MODE"=2114720, "SENSITIVITY"=2114992, "PHOTON IMAGING MODE"=2115200, "HIGH DYNAMIC RANGE MODE"=3163360, "WHITE BALANCE"=3163568, "TEMPERATURE"=2115232, "TEMPERATURE TARGET"=2115264, "SENSOR COOLER FAN"=2115296, "LINEBUNDLE HEIGHT"=4212192, "MECHANICAL SHUTTER"=2115488, "BACK FOCUS POSITION"=8422304, "TRIGGER CONNECTOR"=1066432, "TRIGGER SOURCE"=1066144, "OUTPUT TRIGGER SOURCE"=1852576, "TRIGGER GLOBAL EXPOSURE"=2049680, "FIRST TRIGGER BEHAVIOR"=2049696, "CHANNEL SYNC"=1852352, "READOUT DIRECTION"=4211904, "PRE HSYNC COUNT"=1852704] ("Parameter")
                w226 = 1 items=["Snap", "Sequence"] ("Capture mode")
                n83 = event-data() -> ("NewVal"=w217:dbl)  [unwired: 1 in, 2 out]
                n84 = call <userlib>:"tm_stopcapture_40.vi"("error in (no error)"=w227, "Handle in"=w228) -> ("error out"=w229:errorcluster, "Handle out"=w230:u32)  [unwired: 8 in]
                n85 = call <userlib>:"tm_unpreparecapture_40.vi"("error in (no error)"=w229, "Handle in"=w230) -> ("error out"=w215:errorcluster, "Handle out"=w216:u32)  [unwired: 8 in]
                n86 = call <userlib>:"tm_setparameter_40.vi"("error in (no error)"=w215, "Value in"=w217, "Parameter"=w212, "Handle in"=w216) -> ("error out"=w214:errorcluster, "Handle out"=w213:u32)  [unwired: 6 in]
                n87 = call <userlib>:"tm_getparameter_40.vi"("error in (no error)"=w214, "Parameter"=w212, "Handle in"=w213) -> ("error out"=w220:errorcluster, "Value out"=w219:dbl, "Handle out"=w218:u32)  [unwired: 6 in]
                n88 = local write "SMD"(w219) -> ()
                n89 = call <userlib>:"tm_preparecapture_40.vi"("error in (no error)"=w220, "Capture mode"=w226, "Handle in"=w218) -> ("error out"=w224:errorcluster, "Handle out"=w225:u32)  [unwired: 5 in, 2 out]
                n90 = call <userlib>:"tm_startcapture_40.vi"("error in (no error)"=w224, "Handle in"=w225) -> ("error out"=w223:errorcluster, "Handle out"=w222:u32)  [unwired: 8 in]
              }
              event "Binning": Value Change {
                w253 = u32 4215968 items=["BINNING"=4215968, "BITS PER CHANNEL"=2, "ACTIVE VIEW INDEX"=3, "CCD MODE"=4, "SENSOR MODE"=5, "READOUT MODE"=6, "EXPOSURE TIME"=7, "CONTRAST GAIN"=8, "CONTRAST OFFSET"=9, "LIGHT MODE"=10, "SENSITIVITY"=11, "WHITE BALANCE"=12, "PHOTON IMAGING MODE"=13, "HIGH DYNAMIC RANGE MODE"=14, "TRIGGER SOURCE"=15, "TRIGGER ACTIVE"=16, "TRIGGER MODE"=17, "TRIGGER POLARITY"=18, "TRIGGER GLOBAL EXPOSURE"=19, "FIRST TRIGGER BEHAVIOR"=20, "TRIGGER TIMES"=21, "OUTPUT TRIGGER POLARITY"=22, "OUTPUT TRIGGER DELAY"=23, "OUTPUT TRIGGER PERIOD"=24, "TEMPERATURE"=25, "TEMPERATURE TARGET"=26, "SENSOR COOLER FAN"=27, "MECHANICAL SHUTTER"=28, "BACK FOCUS POSITION"=29, "FRAMEBUNDLE MODE"=30, "FRAMEBUNDLE NUMBER"=31, "LINEBUNDLE HEIGHT"=32, "TRIGGER CONNECTOR"=33, "IMAGE PIXEL TYPE"=34, "OUTPUT TRIGGER KIND"=35, "READOUT DIRECTION"=36, "CHANNEL SYNC"=37] ("Parameter")
                w266 = 1 items=["Snap", "Sequence"] ("Capture mode")
                n91 = event-data() -> ("NewVal"=w251:u16)  [unwired: 1 in, 2 out]
                n92 = call <userlib>:"tm_stopcapture_40.vi"("error in (no error)"=w258, "Handle in"=w259) -> ("error out"=w256:errorcluster, "Handle out"=w257:u32)  [unwired: 8 in]
                n93 = call <userlib>:"tm_unpreparecapture_40.vi"("error in (no error)"=w256, "Handle in"=w257) -> ("error out"=w254:errorcluster, "Handle out"=w252:u32)  [unwired: 8 in]
                n94 = call <userlib>:"tm_setparameter_40.vi"("error in (no error)"=w254, "Value in"=w251, "Parameter"=w253, "Handle in"=w252) -> ("error out"=w248:errorcluster, "Handle out"=w249:u32)  [unwired: 6 in]
                n95 = call <userlib>:"tm_getarea_40.vi"("error in (no error)"=w248, "Handle in"=w249) -> ("error out"=w246:errorcluster, "Sub Region"=w250:T5, "Handle out"=w247:u32)  [unwired: 7 in]
                n96 = Unbundle(w250) -> ("H Offset"=w237:cluster{"Value":i32, "Limits":T4}, "V Offset"=w236:cluster{"Value":i32, "Limits":T4}, "H Size"=w235:cluster{"Value":i32, "Limits":T4}, "V Size"=w234:cluster{"Value":i32, "Limits":T4})
                n97 = Unbundle By Name(w237) -> ("Value"=w245:i32, "Limits"=w244:T4)
                n98 = Unbundle By Name(w236) -> ("Value"=w243:i32, "Limits"=w242:T4)
                n99 = Unbundle By Name(w235) -> ("Value"=w241:i32, "Limits"=w240:T4)
                n100 = Unbundle By Name(w234) -> ("Value"=w239:i32, "Limits"=w238:T4)
                n101 = property on="H Offset" class="DigNum (strict)"("Value"=w245, "Data Range"=w244) -> ()  [unwired: 2 in, 2 out]
                n102 = property on="V Offset" class="DigNum (strict)"("Value"=w243, "Data Range"=w242) -> ()  [unwired: 2 in, 2 out]
                n103 = property on="H Width" class="DigNum (strict)"("Value"=w241, "Data Range"=w240) -> ()  [unwired: 2 in, 2 out]
                n104 = property on="V Width" class="DigNum (strict)"("Value"=w239, "Data Range"=w238) -> ()  [unwired: 2 in, 2 out]
                n105 = local write "SHO"(w245) -> ()
                n106 = local write "SVO"(w243) -> ()
                n107 = local write "SHW"(w241) -> ()
                n108 = local write "SVW"(w239) -> ()
                n109 = call <userlib>:"tm_preparecapture_40.vi"("error in (no error)"=w246, "Capture mode"=w266, "Handle in"=w247) -> ("error out"=w264:errorcluster, "Handle out"=w265:u32)  [unwired: 5 in, 2 out]
                n110 = call <userlib>:"tm_startcapture_40.vi"("error in (no error)"=w264, "Handle in"=w265) -> ("error out"=w263:errorcluster, "Handle out"=w262:u32)  [unwired: 8 in]
              }
              event "H Offset", "H Width", "V Offset", "V Width": Value Change {
                w280 = u32 4215968 items=["SENSOR MODE"=4212128, "READOUT SPEED"=4211872, "READOUT DIRECTION"=4211904, "TRIGGER GLOBAL EXPOSURE"=2049680, "TRIGGER DELAY"=1066480, "INTERNAL TRIGGER HANDLING"=1066496, "SENSOR TEMPERATURE"=2115232, "SENSOR COOLER STATUS"=2115280, "EXPOSURE TIME"=2049184, "DEFECT CORRECT MODE"=4670368, "HOT PIXEL CORRECT LEVEL"=4670400, "BINNING"=4215968, "TIMING READOUT TIME"=4223904, "INTERNAL FRAME RATE"=4225952, "INTERNAL FRAME INTERVAL"=4225968, "INTERNAL LINE SPEED"=4226000, "INTERNAL LINE INTERVAL"=4226016, "IMAGE WIDTH"=4343200, "IMAGE HEIGHT"=4343216, "IMAGE ROWBYTES"=4343232, "IMAGE FRAMEBYTES"=4343248, "IMAGE PIXEL TYPE"=4343296, "NUMBER OF OUTPUT TRIGGER CONNECTOR"=1852320, "OUTPUT TRIGGER SOURCE[0]"=1852576, "OUTPUT TRIGGER SOURCE[1]"=1852832, "OUTPUT TRIGGER SOURCE[2]"=1853088, "OUTPUT TRIGGER POLARITY[0]"=1852592, "OUTPUT TRIGGER POLARITY[1]"=1852848, "OUTPUT TRIGGER POLARITY[2]"=1853104, "OUTPUT TRIGGER ACTIVE[0]"=1852608, "OUTPUT TRIGGER ACTIVE[1]"=1852864, "OUTPUT TRIGGER ACTIVE[2]"=1853120, "OUTPUT TRIGGER DELAY[0]"=1852624, "OUTPUT TRIGGER DELAY[1]"=1852880, "OUTPUT TRIGGER DELAY[2]"=1853136, "OUTPUT TRIGGER PERIOD[0]"=1852640, "OUTPUT TRIGGER PERIOD[1]"=1852896, "OUTPUT TRIGGER PERIOD[2]"=1853152, "OUTPUT TRIGGER KIND[0]"=1852656, "OUTPUT TRIGGER KIND[1]"=1852912, "OUTPUT TRIGGER KIND[2]"=1853168, "OUTPUT TRIGGER BASE SENSOR[0]"=1852672, "OUTPUT TRIGGER BASE SENSOR[1]"=1852928, "OUTPUT TRIGGER BASE SENSOR[2]"=1853184, "OUTPUT TRIGGER PRE HSYNC COUNT"=1852704] ("Parameter")
                w312 = 1 items=["Snap", "Sequence"] ("Capture mode")
                n111 = event-data() -> ()  [unwired: 1 in, 4 out]
                n112 = call <userlib>:"tm_stopcapture_40.vi"("error in (no error)"=w303, "Handle in"=w304) -> ("error out"=w301:errorcluster, "Handle out"=w302:u32)  [unwired: 8 in]
                n113 = local read "H Offset"() -> (w277:i32)
                n114 = local read "H Width"() -> (w275:i32)
                n115 = local read "V Offset"() -> (w276:i32)
                n116 = local read "V Width"() -> (w274:i32)
                n117 = call <userlib>:"tm_unpreparecapture_40.vi"("error in (no error)"=w301, "Handle in"=w302) -> ("error out"=w281:errorcluster, "Handle out"=w282:u32)  [unwired: 8 in]
                n118 = call <userlib>:"tm_getparameter_40.vi"("error in (no error)"=w281, "Parameter"=w280, "Handle in"=w282) -> ("error out"=w278:errorcluster, "Value out"=w269:dbl, "Handle out"=w279:u32)  [unwired: 6 in]
                n119 = To Long Integer(number=w269) -> (32bit integer=w268:i32)
                n120 = Multiply(x=w274, y=w268) -> (x*y=w270:i32)
                n121 = Multiply(x=w275, y=w268) -> (x*y=w271:i32)
                n122 = Multiply(x=w276, y=w268) -> (x*y=w272:i32)
                n123 = Multiply(x=w277, y=w268) -> (x*y=w273:i32)
                n124 = Bundle(w273, w272, w271, w270) -> (w305:cluster{i32, i32, i32, i32})  [unwired: 1 in]
                n125 = call <userlib>:"tm_setarea_40.vi"("error in (no error)"=w278, "Sub Region"=w305, "Handle in"=w279) -> ("error out"=w298:errorcluster, "Handle out"=w299:u32)  [unwired: 7 in]
                n126 = call <userlib>:"tm_getarea_40.vi"("error in (no error)"=w298, "Handle in"=w299) -> ("error out"=w296:errorcluster, "Sub Region"=w288:T5, "Handle out"=w297:u32)  [unwired: 7 in]
                n127 = Unbundle(w288) -> ("H Offset"=w295:cluster{"Value":i32, "Limits":T4}, "V Offset"=w294:cluster{"Value":i32, "Limits":T4}, "H Size"=w293:cluster{"Value":i32, "Limits":T4}, "V Size"=w292:cluster{"Value":i32, "Limits":T4})
                n128 = Unbundle By Name(w295) -> ("Value"=w291:i32, "Limits"=w290:T4)
                n129 = Unbundle By Name(w294) -> ("Value"=w289:i32, "Limits"=w284:T4)
                n130 = Unbundle By Name(w293) -> ("Value"=w285:i32, "Limits"=w283:T4)
                n131 = Unbundle By Name(w292) -> ("Value"=w287:i32, "Limits"=w286:T4)
                n132 = property on="H Offset" class="DigNum (strict)"("Value"=w291, "Data Range"=w290) -> ()  [unwired: 2 in, 2 out]
                n133 = property on="V Offset" class="DigNum (strict)"("Value"=w289, "Data Range"=w284) -> ()  [unwired: 2 in, 2 out]
                n134 = property on="H Width" class="DigNum (strict)"("Value"=w285, "Data Range"=w283) -> ()  [unwired: 2 in, 2 out]
                n135 = property on="V Width" class="DigNum (strict)"("Value"=w287, "Data Range"=w286) -> ()  [unwired: 2 in, 2 out]
                n136 = call <userlib>:"tm_preparecapture_40.vi"("error in (no error)"=w296, "Capture mode"=w312, "Handle in"=w297) -> ("error out"=w310:errorcluster, "Handle out"=w311:u32)  [unwired: 5 in, 2 out]
                n137 = local write "SHO"(w291) -> ()
                n138 = local write "SVO"(w289) -> ()
                n139 = local write "SHW"(w285) -> ()
                n140 = local write "SVW"(w287) -> ()
                n141 = call <userlib>:"tm_startcapture_40.vi"("error in (no error)"=w310, "Handle in"=w311) -> ("error out"=w309:errorcluster, "Handle out"=w308:u32)  [unwired: 8 in]
              }
            }
            n142 = Unbundle By Name(w130) -> ("status"=w142:bool)
            n143 = Or(x=w142, y="stop") -> (x .or. y?=w141:bool)
          }
          n144 = call <userlib>:"tm_stopcapture_40.vi"("error in (no error)"=w112, "Handle in"=w113) -> ("error out"=w109:errorcluster, "Handle out"=w110:u32)  [unwired: 8 in]
          n145 = call <userlib>:"tm_unpreparecapture_40.vi"("error in (no error)"=w109, "Handle in"=w110) -> ("error out"=w108:errorcluster, "Handle out"=w111:u32)  [unwired: 8 in]
          n146 = call <userlib>:"tm_closecamera_40.vi"("error in (no error)"=w108, "Handle in"=w111) -> ("error out"=w122:errorcluster)  [unwired: 9 in]
          n147 = call <userlib>:"tm_deinitialize_40.vi"("error in (no error)"=w122) -> ("error out"=w121:errorcluster)  [unwired: 10 in]
        }
      }
      "error out" <- w45
      n148 = while {
        tunnel: w70 -> [w945]
        tunnel: [w944] -> w68
        tunnel: w69 -> [w943]
        tunnel: [w942] -> w67
        tunnel: w66 -> [w940]
        shift-right: [w884] -> _
        shift-left: _ -> [w883]
        stop <- FALSE stop-if-true
        (unwired) 200000.0 ("y")
        n149 = Tick Count (ms)() -> (millisecond timer value=w939:u32)
        n150 = Subtract(x=w939, y=w940) -> (x-y=w934:u32)
        n151 = Divide(x="Threshold1", y="ratiocontrol") -> (x/y=w927:dbl)
        n152 = Divide(x="Threshold2", y="ratiocontrol") -> (x/y=w926:dbl)
        n153 = Multiply(x="determine ratio (xx.xx)", y=100.0) -> (x*y=w907:dbl)
        n154 = Multiply(x="Droplet width [ms]", y=0.001) -> (x*y=w909:dbl)
        n155 = Multiply(x=0.001, y=w934) -> (x*y=w901:dbl)
        "LabView Timer (sec)" <- w901
        n156 = Quotient & Remainder(x=w934, y=u32 1) -> (x-y*floor(x/y)=w936:u32)  [unwired: 1 out]
        n157 = Multiply(x=w909, y=w883) -> (x*y=w908:dbl)
        n158 = To Unsigned Quad Integer(1:w908) -> (0:w922:u64)
        n159 = xnode "Read/Write Control"("FPGA VI Reference In"=w945, "error in"=w943, "Threshold1"=w927, "Threshold2"=w926, "Time compensation [clock]"=w922, "FPGA initializer"="FPGA initializer", "determine ratio"=w907) -> ("FPGA VI Reference Out"=w944:refnum<k20>, "error out"=w942:errorcluster, "Sort"=w925:bool, "Unfiltered  Signal1"=w904:i16, "Filtered Signal1"=w892:i16, "Unfiltered  Signal2"=w928:i16, "Filtered Signal2"=w903:i16, "t0 (sample)"=→"t0 (sample)":u64, "t1 (sample)"=→"t1 (sample)":u64, "Droplet counter"=→"Droplet counter":u64, "Sorted droplet counter"=→"Sorted droplet counter":u64, "loop counter"=w913:u64, "Droplet lock on"=→"Droplet lock on":bool, "PMT1 sum"=w886:u64, "PMT2 sum"=w885:u64, "sample diff"=→"sample diff":u64, "Loop length (uSec)"=w912:u32)  [unwired: 1 out]
        "Unfiltered Signal 1" <- w904
        "Filtered Signal 2" <- w903
        "Unfiltered Signal 2" <- w928
        "PMT1 sum" <- w886
        "PMT2 sum" <- w885
        "FPGA loop counter" <- w913
        "Sort" <- w925
        "Filtered Signal 1" <- w892
        "PMT1 sum" <- w886
        "PMT2 sum" <- w885
        n160 = case shown="0" w936 {
          tunnel: w928 -> [_ w961]
          tunnel: w903 -> [_ w960]
          tunnel: w892 -> [_ w959]
          tunnel: w904 -> [_ w958]
          tunnel: w926 -> [_ w956]
          tunnel: w927 -> [_ w955]
          tunnel: w925 -> [_ w953]
          tunnel: w901 -> [_ w951]
          tunnel: "ratiocontrol" -> [_ w949]
          frame Default {
          }
          frame 0 {
            n161 = Number To Fractional String(number=w951) -> (F-format string=w950:string)  [unwired: 3 in]
            n162 = Format Into String(w955) -> (resulting string=w963:string)  [unwired: 3 in, 1 out]
            n163 = Multiply(x=w958, y=w949) -> (x*y=w971:dbl)
            n164 = Format Into String(w971) -> (resulting string=w962:string)  [unwired: 3 in, 1 out]
            n165 = Multiply(x=w959, y=w949) -> (x*y=w972:dbl)
            n166 = Format Into String(w956) -> (resulting string=w965:string)  [unwired: 3 in, 1 out]
            n167 = Format Into String(w972) -> (resulting string=w964:string)  [unwired: 3 in, 1 out]
            n168 = Format Into String(w953) -> (resulting string=w952:string)  [unwired: 3 in, 1 out]
            n169 = Multiply(x=w961, y=w949) -> (x*y=w973:dbl)
            n170 = Format Into String(w973) -> (resulting string=w966:string)  [unwired: 3 in, 1 out]
            n171 = Multiply(x=w960, y=w949) -> (x*y=w974:dbl)
            n172 = Format Into String(w974) -> (resulting string=w967:string)  [unwired: 3 in, 1 out]
            n173 = Build Array(w963, w962, w964, w952, w950, "" ("element"), w965, w966, w967, w952, w950) -> (w969:string[])
            n174 = Array To Spreadsheet String(array=w969, 3:"%s" ("format string")) -> (spreadsheet string=w968:string)  [unwired: 1 in]
            n175 = local read "Data File Ptr"() -> (w970:refnum<file>)
            n176 = Write to Text File(file (use dialog)=w970, text=w968) -> ()  [unwired: 2 in, 3 out]
          }
        }
        n177 = To Double Precision Float(number=w886) -> (double precision float=w891:dbl)
        n178 = To Double Precision Float(number=w885) -> (double precision float=w890:dbl)
        n179 = Divide(x=w891, y=w890) -> (x/y=w887:dbl)
        n180 = Not A Number/Path/Refnum?(number/path/refnum=w887) -> (NaN/Path/Refnum?=w889:bool)
        n181 = case shown="False" w889 {
          tunnel: [w946 0.0] -> w888
          tunnel: w887 -> [w946 _]
          frame False {
          }
          frame True {
          }
        }
        "PMT1/PMT2" <- w888
        "PMT1/PMT2 (graph)" <- w888
        n182 = Multiply(x="ratiocontrol", y=w904) -> (x*y=→"Unfiltered Signal1":dbl)
        n183 = Divide(x=w912, y=1000000.0 ("x")) -> (x/y=w910:dbl)
        n184 = call "Tick Count"() -> ("Tick Count(uSec)"=w894:u32)
        n185 = Divide(x=1.0, y=w910) -> (x/y=w884:dbl)
        "FPGA freq" <- w884
        n186 = local read "FPGA initializer"() -> (w914:bool)
        n187 = Divide(x=w913, y=w884) -> (x/y=→"FPGA timer (sec)":dbl)
        n188 = feedback #1() -> (w893:u32)  [unwired: 1 in]
        n189 = feedback-in #1(w894) -> ()
        n190 = Multiply(x="ratiocontrol", y=w892) -> (x*y=→"Filtered Signal1":dbl)
        n191 = Subtract(x=w894, y=w893) -> (x-y=w895:u32)
        n192 = case shown="True" w914 {
          frame False {
          }
          frame True {
            n193 = local write "FPGA initializer"(FALSE ("FPGA initializer")) -> ()
          }
        }
        n194 = Multiply(x="ratiocontrol", y=w928) -> (x*y=→"Unfiltered Signal2":dbl)
        n195 = Divide(x=w895, y=1000000.0 ("x")) -> (x/y=w898:dbl)
        n196 = Multiply(x="ratiocontrol", y=w903) -> (x*y=→"Filtered Signal2":dbl)
        n197 = Divide(x=1.0, y=w898) -> (x/y=→"LabView freq":dbl)
      }
      n198 = while {
        shift-right: [w314] -> w47
        shift-left: w50 -> [w402]
        shift-right: [w317] -> w51
        shift-left: w49 -> [w401]
        shift-right: [w315] -> _
        shift-left: _ -> [w399]
        stop <- "Arduino \nshut down" continue-if-true
        n199 = case shown="False" "Initializer" {
          tunnel: w402 -> [w519 w529]
          tunnel: w401 -> [w520 w528]
          tunnel: [w519 w525] -> w398
          tunnel: [w520 w524] -> w397
          tunnel: w399 -> [w521 w523]
          tunnel: [w521 w523] -> w396
          frame False {
          }
          frame True {
            n200 = local write "Initializer"(FALSE ("send")) -> ()
            n201 = Wait (ms)(milliseconds to wait=u32 100) -> ()  [unwired: 1 out]
            n202 = VISA Write(VISA resource name=w529, write buffer="LV_INIT", error in (no error)=w528) -> (VISA resource name out=w525:refnum<visa-resource-name>, error out=w524:errorcluster)  [unwired: 1 out]
          }
        }
        n203 = Divide(x="PMT1 senstivity input", y=5.0) -> (x/y=w368:dbl)
        n204 = Multiply(x=w368, y=128.0) -> (x*y=w370:dbl)
        n205 = Subtract(x=w370, y=1.0) -> (x-y=w365:dbl)
        n206 = Round To Nearest(number=w365) -> (nearest integer value=w374:dbl)
        n207 = Format Into String(w374) -> (resulting string=w373:string)  [unwired: 3 in, 1 out]
        n208 = Concatenate Strings("POT1 " ("string"), w373) -> (w371:string)
        n209 = Divide(x="PMT2 senstivity input", y=5.0) -> (x/y=w360:dbl)
        n210 = case shown="False" "PMT1 senstivity" {
          tunnel: w398 -> [w509 w518]
          tunnel: w397 -> [w508 w517]
          tunnel: [w509 w514] -> w395
          tunnel: [w508 w513] -> w394
          tunnel: w396 -> [w510 w512]
          tunnel: [w510 w512] -> w393
          tunnel: w371 -> [_ w511]
          frame False {
          }
          frame True {
            n211 = VISA Write(VISA resource name=w518, write buffer=w511, error in (no error)=w517) -> (VISA resource name out=w514:refnum<visa-resource-name>, error out=w513:errorcluster)  [unwired: 1 out]
            n212 = local write "PMT1 senstivity"(FALSE ("send")) -> ()
            n213 = Wait (ms)(milliseconds to wait=u32 100) -> ()  [unwired: 1 out]
          }
        }
        n214 = Multiply(x=w360, y=128.0) -> (x*y=w358:dbl)
        n215 = Subtract(x=w358, y=1.0) -> (x-y=w362:dbl)
        n216 = Round To Nearest(number=w362) -> (nearest integer value=w355:dbl)
        n217 = Format Into String(w355) -> (resulting string=w356:string)  [unwired: 3 in, 1 out]
        n218 = Concatenate Strings("POT2 " ("string"), w356) -> (w353:string)
        n219 = case shown="False" "PMT2 senstivity" {
          tunnel: w395 -> [w497 w507]
          tunnel: w394 -> [w498 w506]
          tunnel: [w497 w503] -> w382
          tunnel: [w498 w502] -> w381
          tunnel: w393 -> [w499 w501]
          tunnel: [w499 w501] -> w383
          tunnel: w353 -> [_ w500]
          frame False {
          }
          frame True {
            n220 = VISA Write(VISA resource name=w507, write buffer=w500, error in (no error)=w506) -> (VISA resource name out=w503:refnum<visa-resource-name>, error out=w502:errorcluster)  [unwired: 1 out]
            n221 = local write "PMT2 senstivity"(FALSE ("send")) -> ()
            n222 = Wait (ms)(milliseconds to wait=u32 100) -> ()  [unwired: 1 out]
          }
        }
        n223 = Divide(x="Func amp input", y=5.0) -> (x/y=w347:dbl)
        n224 = Multiply(x=w347, y=128.0) -> (x*y=w349:dbl)
        n225 = Subtract(x=w349, y=1.0) -> (x-y=w345:dbl)
        n226 = Round To Nearest(number=w345) -> (nearest integer value=w351:dbl)
        n227 = Format Into String(w351) -> (resulting string=w350:string)  [unwired: 3 in, 1 out]
        n228 = Concatenate Strings("POT_HV AMP " ("string"), w350) -> (w343:string)
        n229 = case shown="False" "Func amp" {
          tunnel: w382 -> [w488 w496]
          tunnel: w381 -> [w486 w495]
          tunnel: [w488 w492] -> w392
          tunnel: [w486 w491] -> w391
          tunnel: w383 -> [w487 w490]
          tunnel: [w487 w490] -> w390
          tunnel: w343 -> [_ w489]
          frame False {
          }
          frame True {
            n230 = VISA Write(VISA resource name=w496, write buffer=w489, error in (no error)=w495) -> (VISA resource name out=w492:refnum<visa-resource-name>, error out=w491:errorcluster)  [unwired: 1 out]
            n231 = local write "Func amp"(FALSE ("send")) -> ()
            n232 = Wait (ms)(milliseconds to wait=u32 100) -> ()  [unwired: 1 out]
          }
        }
        n233 = Format Into String("Func freq input") -> (resulting string=w342:string)  [unwired: 3 in, 1 out]
        n234 = Concatenate Strings("POT_HV FRQ " ("string"), w342) -> (w339:string)
        n235 = case shown="False" "Func Freq" {
          tunnel: w392 -> [w476 w485]
          tunnel: w391 -> [w475 w484]
          tunnel: [w476 w481] -> w384
          tunnel: [w475 w480] -> w385
          tunnel: w390 -> [w477 w479]
          tunnel: [w477 w479] -> w389
          tunnel: w339 -> [_ w478]
          frame False {
          }
          frame True {
            n236 = VISA Write(VISA resource name=w485, write buffer=w478, error in (no error)=w484) -> (VISA resource name out=w481:refnum<visa-resource-name>, error out=w480:errorcluster)  [unwired: 1 out]
            n237 = local write "Func Freq"(FALSE ("send")) -> ()
            n238 = Wait (ms)(milliseconds to wait=u32 100) -> ()  [unwired: 1 out]
          }
        }
        n239 = Multiply(x="Func on Time input", y=1000.0) -> (x*y=w329:dbl)
        n240 = Format Into String(w329) -> (resulting string=w338:string)  [unwired: 3 in, 1 out]
        n241 = Concatenate Strings("POT_HV ONT " ("string"), w338) -> (w337:string)
        n242 = case shown="False" "Func On time" {
          tunnel: w385 -> [w464 w474]
          tunnel: [w465 w471] -> w387
          tunnel: [w464 w470] -> w386
          tunnel: w389 -> [w466 w469]
          tunnel: [w466 w469] -> w388
          tunnel: w384 -> [w465 w468]
          tunnel: w337 -> [_ w467]
          frame False {
          }
          frame True {
            n243 = VISA Write(VISA resource name=w468, write buffer=w467, error in (no error)=w474) -> (VISA resource name out=w471:refnum<visa-resource-name>, error out=w470:errorcluster)  [unwired: 1 out]
            n244 = local write "Func On time"(FALSE ("send")) -> ()
            n245 = Wait (ms)(milliseconds to wait=u32 100) -> ()  [unwired: 1 out]
          }
        }
        n246 = Multiply(x="Func delay input", y=1000.0) -> (x*y=w327:dbl)
        n247 = Format Into String(w327) -> (resulting string=w336:string)  [unwired: 3 in, 1 out]
        n248 = Concatenate Strings("POT_HV DLY " ("string"), w336) -> (w335:string)
        n249 = case shown="True" "Func Delay" {
          tunnel: w387 -> [w455 w463]
          tunnel: w386 -> [w454 w462]
          tunnel: [w455 w459] -> w319
          tunnel: [w454 w458] -> w318
          tunnel: w388 -> [w453 w457]
          tunnel: [w453 w457] -> w316
          tunnel: w335 -> [_ w456]
          frame False {
          }
          frame True {
            n250 = VISA Write(VISA resource name=w463, write buffer=w456, error in (no error)=w462) -> (VISA resource name out=w459:refnum<visa-resource-name>, error out=w458:errorcluster)  [unwired: 1 out]
            n251 = local write "Func Delay"(FALSE ("send")) -> ()
            n252 = Wait (ms)(milliseconds to wait=u32 100) -> ()  [unwired: 1 out]
          }
        }
        n253 = feedback #2(FALSE ("Motor Start/Stop")) -> (w323:bool)
        n254 = feedback-in #2("Merger on") -> ()
        n255 = Build Array("Merger on", w323) -> (w322:bool[])
        n256 = Boolean Array To Number(Boolean array=w322) -> (number=w325:u32)
        n257 = case shown="1" w325 {
          tunnel: "MERGE " ("string") -> [_ w418 w438]
          tunnel: w316 -> [_ w413 w436]
          tunnel: [w408 w414 w435] -> w314
          tunnel: [w404 w413 w436] -> w315
          tunnel: [w407 w415 w437] -> w317
          tunnel: w318 -> [w406 w416 w434]
          tunnel: w319 -> [w405 w417 w433]
          frame 0, Default {
            n258 = Wait (ms)(milliseconds to wait=u32 100) -> ()  [unwired: 1 out]
            n259 = property class="Instr"(reference=w405, error in=w406) -> (reference out=w411:refnum<visa-resource-name>, error out=w409:errorcluster, "Bytes at Port"=w410:u32)
            n260 = VISA Read(VISA resource name=w411, byte count=w410, error in (no error)=w409) -> (VISA resource name out=w408:refnum<visa-resource-name>, read buffer=w404:string, error out=w407:errorcluster)  [unwired: 1 out]
            "Serial debugger" <- w404
          }
          frame 1 {
            n261 = Concatenate Strings(w418, "ON " ("string")) -> (w421:string)
            n262 = flat-sequence {
              tunnel: w421 -> [w428]
              tunnel: w417 -> [w427]
              tunnel: w416 -> [w426]
              tunnel: [w425] -> w420
              tunnel: [w424] -> w419
              tunnel: w420 -> [w432]
              tunnel: w419 -> [w431]
              tunnel: [w430] -> w414
              tunnel: [w429] -> w415
              frame #0 {
                n263 = VISA Write(VISA resource name=w427, write buffer=w428, error in (no error)=w426) -> (VISA resource name out=w425:refnum<visa-resource-name>, error out=w424:errorcluster)  [unwired: 1 out]
                n264 = Wait Until Next ms Multiple(millisecond multiple=u32 100) -> ()  [unwired: 1 out]
              }
              frame #1 {
                n265 = VISA Clear(VISA resource name=w432, error in (no error)=w431) -> (VISA resource name out=w430:refnum<visa-resource-name>, error out=w429:errorcluster)
              }
            }
          }
          frame 2 {
            n266 = Concatenate Strings(w438, "OFF " ("string")) -> (w441:string)
            n267 = flat-sequence {
              tunnel: w441 -> [w448]
              tunnel: w433 -> [w445]
              tunnel: w434 -> [w444]
              tunnel: [w447] -> w440
              tunnel: [w446] -> w439
              tunnel: [w452] -> w437
              tunnel: [w449] -> w435
              tunnel: w440 -> [w451]
              tunnel: w439 -> [w450]
              frame #0 {
                n268 = VISA Write(VISA resource name=w445, write buffer=w448, error in (no error)=w444) -> (VISA resource name out=w447:refnum<visa-resource-name>, error out=w446:errorcluster)  [unwired: 1 out]
                n269 = Wait Until Next ms Multiple(millisecond multiple=u32 100) -> ()  [unwired: 1 out]
              }
              frame #1 {
                n270 = VISA Clear(VISA resource name=w451, error in (no error)=w450) -> (VISA resource name out=w449:refnum<visa-resource-name>, error out=w452:errorcluster)
              }
            }
          }
        }
      }
      n271 = while {
        shift-right: [w535] -> w56
        shift-left: w59 -> [w537]
        shift-right: [w534] -> w55
        shift-left: w58 -> [w536]
        stop <- "Shut down program" continue-if-true
        w574 = "2" ("trimmed string")
        w579 = "1" ("trimmed string")
        w593 = "3" ("trimmed string")
        n272 = case shown="\"CUS\"" "Syringe Selection1" {
          tunnel: ["dia1 (mm)" 4.699 ("dia (mm)") 8.66 ("dia (mm)") 12.07 ("dia (mm)") 14.5 ("dia (mm)") w754] -> w614
          frame "CUS" {
            n273 = property on="dia1 (mm)" class="DigNum (strict)"("DisabledEnum"=T2."Enabled" ("Disabled")) -> ()  [unwired: 2 in, 2 out]
          }
          frame "BDP1MM" {
            n274 = property on="dia1 (mm)" class="DigNum (strict)"("DisabledEnum"=T2."Disabled and Grayed Out" ("Disabled")) -> ()  [unwired: 2 in, 2 out]
          }
          frame "BDP3MM" {
            n275 = property on="dia1 (mm)" class="DigNum (strict)"("DisabledEnum"=T2."Disabled and Grayed Out" ("Disabled")) -> ()  [unwired: 2 in, 2 out]
          }
          frame "BDP5MM" {
            n276 = property on="dia1 (mm)" class="DigNum (strict)"("DisabledEnum"=T2."Disabled and Grayed Out" ("Disabled")) -> ()  [unwired: 2 in, 2 out]
          }
          frame "BDP10MM" {
            n277 = property on="dia1 (mm)" class="DigNum (strict)"("DisabledEnum"=T2."Disabled and Grayed Out" ("Disabled")) -> ()  [unwired: 2 in, 2 out]
          }
          frame Default {
            n278 = property on="dia1 (mm)" class="DigNum (strict)"("DisabledEnum"=T2."Enabled" ("Disabled")) -> ()  [unwired: 2 in, 2 out]
            n279 = property on="dia1 (mm)" class="DigNum (strict)"() -> ("Value"=w754:dbl)  [unwired: 2 in, 2 out]
          }
        }
        "Diameter1 (mm)" <- w614
        n280 = feedback #3(FALSE ("Go 1")) -> (w628:bool)
        n281 = feedback-in #3("Send1") -> ()
        n282 = case shown="\"BDP10MM\"" "Syringe Selection2" {
          tunnel: ["dia2 (mm)" 4.78 ("dia (mm)") 8.66 ("dia (mm)") 12.07 ("dia (mm)") 14.5 ("dia (mm)") w729] -> w606
          frame "CUS" {
            n283 = property on="dia2 (mm)" class="DigNum (strict)"("DisabledEnum"=T2."Enabled" ("Disabled")) -> ()  [unwired: 2 in, 2 out]
          }
          frame "BDP1MM" {
            n284 = property on="dia2 (mm)" class="DigNum (strict)"("DisabledEnum"=T2."Disabled and Grayed Out" ("Disabled")) -> ()  [unwired: 2 in, 2 out]
          }
          frame "BDP3MM" {
            n285 = property on="dia2 (mm)" class="DigNum (strict)"("DisabledEnum"=T2."Disabled and Grayed Out" ("Disabled")) -> ()  [unwired: 2 in, 2 out]
          }
          frame "BDP5MM" {
            n286 = property on="dia2 (mm)" class="DigNum (strict)"("DisabledEnum"=T2."Disabled and Grayed Out" ("Disabled")) -> ()  [unwired: 2 in, 2 out]
          }
          frame "BDP10MM" {
            n287 = property on="dia2 (mm)" class="DigNum (strict)"("DisabledEnum"=T2."Disabled and Grayed Out" ("Disabled")) -> ()  [unwired: 2 in, 2 out]
          }
          frame Default {
            n288 = property on="dia2 (mm)" class="DigNum (strict)"("DisabledEnum"=T2."Enabled" ("Disabled")) -> ()  [unwired: 2 in, 2 out]
            n289 = property on="dia2 (mm)" class="DigNum (strict)"() -> ("Value"=w729:dbl)  [unwired: 2 in, 2 out]
          }
        }
        "Diameter2 (mm)" <- w606
        n290 = formula code="r=p*((d/20)**2)*5.1;"("d"=w614, "p"=3.141592653589793) -> ("r"=w633:dbl)
        n291 = case shown="\"mm\"" "Units1" {
          tunnel: w633 -> [w766 w768 w772 w776 w777]
          tunnel: [w765 w769 w771 w776 w777] -> w634
          frame "mh" {
            n292 = Multiply(x=w766, y=60.0) -> (x*y=w765:dbl)
          }
          frame "um" {
            n293 = Multiply(x=1000.0, y=w768) -> (x*y=w769:dbl)
          }
          frame "uh" {
            n294 = Multiply(x=1000.0, y=60.0) -> (x*y=w775:dbl)
            n295 = Multiply(x=w775, y=w772) -> (x*y=w771:dbl)
          }
          frame Default {
          }
          frame "mm" {
          }
        }
        "Max rate1" <- w634
        n296 = case shown="Default" "Syringe Selection3" {
          tunnel: ["dia3 (mm)" 4.78 ("dia (mm)") 8.66 ("dia (mm)") 12.07 ("dia (mm)") 14.5 ("dia (mm)") w704] -> w596
          frame "CUS" {
            n297 = property on="dia3 (mm)" class="DigNum (strict)"("DisabledEnum"=T2."Enabled" ("Disabled")) -> ()  [unwired: 2 in, 2 out]
          }
          frame "BDP1MM" {
            n298 = property on="dia3 (mm)" class="DigNum (strict)"("DisabledEnum"=T2."Disabled and Grayed Out" ("Disabled")) -> ()  [unwired: 2 in, 2 out]
          }
          frame "BDP3MM" {
            n299 = property on="dia3 (mm)" class="DigNum (strict)"("DisabledEnum"=T2."Disabled and Grayed Out" ("Disabled")) -> ()  [unwired: 2 in, 2 out]
          }
          frame "BDP5MM" {
            n300 = property on="dia3 (mm)" class="DigNum (strict)"("DisabledEnum"=T2."Disabled and Grayed Out" ("Disabled")) -> ()  [unwired: 2 in, 2 out]
          }
          frame "BDP10MM" {
            n301 = property on="dia3 (mm)" class="DigNum (strict)"("DisabledEnum"=T2."Disabled and Grayed Out" ("Disabled")) -> ()  [unwired: 2 in, 2 out]
          }
          frame Default {
            n302 = property on="dia3 (mm)" class="DigNum (strict)"("DisabledEnum"=T2."Enabled" ("Disabled")) -> ()  [unwired: 2 in, 2 out]
            n303 = property on="dia3 (mm)" class="DigNum (strict)"() -> ("Value"=w704:dbl)  [unwired: 2 in, 2 out]
          }
        }
        "Diameter3 (mm)" <- w596
        n304 = formula code="r=p*((d/20)**2)*5.1;"("d"=w596, "p"=3.141592653589793) -> ("r"=w598:dbl)
        n305 = case shown="\"uh\"" "Units3" {
          tunnel: w598 -> [w706 w708 w712 w716 w717]
          tunnel: [w705 w709 w711 w716 w717] -> w599
          frame "mh" {
            n306 = Multiply(x=w706, y=60.0) -> (x*y=w705:dbl)
          }
          frame "um" {
            n307 = Multiply(x=1000.0, y=w708) -> (x*y=w709:dbl)
          }
          frame "uh" {
            n308 = Multiply(x=1000.0, y=60.0) -> (x*y=w715:dbl)
            n309 = Multiply(x=w715, y=w712) -> (x*y=w711:dbl)
          }
          frame Default {
          }
          frame "mm" {
          }
        }
        "Max rate3" <- w599
        n310 = formula code="r=p*((d/20)**2)*5.1;"("d"=w606, "p"=3.141592653589793) -> ("r"=w608:dbl)
        n311 = Or(x="Send1", y=w628) -> ()  [unwired: 1 out]
        n312 = case shown="\"mh\"" "Units2" {
          tunnel: w608 -> [w731 w733 w737 w741 w742]
          tunnel: [w730 w734 w736 w741 w742] -> w609
          frame "mh" {
            n313 = Multiply(x=w731, y=60.0) -> (x*y=w730:dbl)
          }
          frame "um" {
            n314 = Multiply(x=1000.0, y=w733) -> (x*y=w734:dbl)
          }
          frame "uh" {
            n315 = Multiply(x=1000.0, y=60.0) -> (x*y=w740:dbl)
            n316 = Multiply(x=w740, y=w737) -> (x*y=w736:dbl)
          }
          frame Default {
          }
          frame "mm" {
          }
        }
        "Max rate2" <- w609
        n317 = Build Array("Send1", w628) -> (w631:bool[])
        n318 = Boolean Array To Number(Boolean array=w631) -> (number=w629:u32)
        n319 = Multiply(x=w634, y=1.3744e-05) -> (x*y=→"Min rate1":dbl)
        n320 = Multiply(x=w609, y=1.3744e-05) -> (x*y=→"Min rate2":dbl)
        n321 = Multiply(x=w599, y=1.3744e-05) -> (x*y=→"Min rate3":dbl)
        n322 = case shown="2" w629 {
          tunnel: w537 -> [w804 w876 w879 w880]
          tunnel: w536 -> [w805 w877 w878 w881]
          tunnel: [w779 w877 w878 w881] -> w592
          tunnel: [w778 w876 w879 w880] -> w591
          tunnel: w614 -> [w801 _ _ _]
          tunnel: "Set rate1" -> [w800 _ _ _]
          tunnel: "Units1" -> [w803 _ _ _]
          tunnel: "Target Vol1" -> [w802 _ _ _]
          tunnel: "Direction1" -> [w806 _ _ _]
          tunnel: w606 -> [w796 _ _ _]
          tunnel: "Set rate2" -> [w795 _ _ _]
          tunnel: "Units2" -> [w792 _ _ _]
          tunnel: "Target Vol2" -> [w791 _ _ _]
          tunnel: "Direction2" -> [w790 _ _ _]
          tunnel: w596 -> [w784 _ _ _]
          tunnel: "Set rate3" -> [w780 _ _ _]
          tunnel: "Units3" -> [w781 _ _ _]
          tunnel: "Direction3" -> [w783 _ _ _]
          tunnel: "Target Vol3" -> [w782 _ _ _]
          tunnel: "Pump1\nStart/Stop" -> [w799 _ _ _]
          tunnel: "Pump2\nStart/Stop" -> [w797 _ _ _]
          tunnel: "Pump3\nStart/Stop" -> [w787 _ _ _]
          frame 2 {
            n323 = case shown="False" w799 {
              tunnel: w806 -> [w854 w870]
              tunnel: w805 -> [w862 w875]
              tunnel: w804 -> [w857 w874]
              tunnel: w803 -> [w856 w871]
              tunnel: w802 -> [w855 w865]
              tunnel: w801 -> [w859 w869]
              tunnel: w800 -> [w858 w867]
              tunnel: [w861 w872] -> w794
              tunnel: [w860 w873] -> w793
              tunnel: "3" ("Pump Add") -> [w853 w863]
              frame True {
                n324 = call "Function_SyringeSetupAssay.vi"("PumpID"=w853, "Diameter (mm)"=w859, "VISA resource name in"=w857, "error in"=w862, "Direction"=w854, "Target Vol1"=w855, "Units"=w856, "Set rate"=w858) -> ("VISA resource name out"=w860:refnum<visa-resource-name>, "error out"=w861:errorcluster)  [unwired: 2 in]
              }
              frame False {
                n325 = Number To Fractional String(number=w869) -> (F-format string=w868:string)  [unwired: 3 in]
                n326 = Number To Fractional String(number=w865) -> (F-format string=w864:string)  [unwired: 3 in]
                n327 = Number To Fractional String(number=w867) -> (F-format string=w866:string)  [unwired: 3 in]
                n328 = call "Function_syringeSetting.vi"("Direction"=w870, "target volume- string"=w864, "error in"=w875, "VISA resource name in"=w874, "units"=w871, "set rate- string"=w866, "diameter(mm)-string"=w868, "address (string)"=w863) -> ("error out"=w872:errorcluster, "VISA resource name out"=w873:refnum<visa-resource-name>)  [unwired: 2 in]
              }
            }
            n329 = case shown="True" w797 {
              tunnel: w790 -> [w831 w847]
              tunnel: w794 -> [w839 w852]
              tunnel: w793 -> [w834 w851]
              tunnel: w792 -> [w833 w848]
              tunnel: w791 -> [w832 w842]
              tunnel: w796 -> [w836 w846]
              tunnel: w795 -> [w835 w844]
              tunnel: [w838 w849] -> w785
              tunnel: [w837 w850] -> w786
              tunnel: "1" ("Pump Add") -> [w830 w840]
              frame True {
                n330 = call "Function_SyringeSetupAssay.vi"("PumpID"=w830, "Diameter (mm)"=w836, "VISA resource name in"=w834, "error in"=w839, "Direction"=w831, "Target Vol1"=w832, "Units"=w833, "Set rate"=w835) -> ("VISA resource name out"=w837:refnum<visa-resource-name>, "error out"=w838:errorcluster)  [unwired: 2 in]
              }
              frame False {
                n331 = Number To Fractional String(number=w842) -> (F-format string=w841:string)  [unwired: 3 in]
                n332 = Number To Fractional String(number=w846) -> (F-format string=w845:string)  [unwired: 3 in]
                n333 = Number To Fractional String(number=w844) -> (F-format string=w843:string)  [unwired: 3 in]
                n334 = call "Function_syringeSetting.vi"("Direction"=w847, "target volume- string"=w841, "error in"=w852, "VISA resource name in"=w851, "units"=w848, "set rate- string"=w843, "diameter(mm)-string"=w845, "address (string)"=w840) -> ("error out"=w849:errorcluster, "VISA resource name out"=w850:refnum<visa-resource-name>)  [unwired: 2 in]
              }
            }
            n335 = case shown="True" w787 {
              tunnel: w783 -> [w808 w825]
              tunnel: w785 -> [w816 w829]
              tunnel: w786 -> [w811 w817]
              tunnel: w781 -> [w810 w826]
              tunnel: w782 -> [w809 w820]
              tunnel: w784 -> [w813 w824]
              tunnel: w780 -> [w812 w822]
              tunnel: [w815 w827] -> w779
              tunnel: [w814 w828] -> w778
              tunnel: "2" ("Pump Add") -> [w807 w818]
              frame True {
                n336 = call "Function_SyringeSetupAssay.vi"("PumpID"=w807, "Diameter (mm)"=w813, "VISA resource name in"=w811, "error in"=w816, "Direction"=w808, "Target Vol1"=w809, "Units"=w810, "Set rate"=w812) -> ("VISA resource name out"=w814:refnum<visa-resource-name>, "error out"=w815:errorcluster)  [unwired: 2 in]
              }
              frame False {
                n337 = Number To Fractional String(number=w820) -> (F-format string=w819:string)  [unwired: 3 in]
                n338 = Number To Fractional String(number=w824) -> (F-format string=w823:string)  [unwired: 3 in]
                n339 = Number To Fractional String(number=w822) -> (F-format string=w821:string)  [unwired: 3 in]
                n340 = call "Function_syringeSetting.vi"("Direction"=w825, "target volume- string"=w819, "error in"=w829, "VISA resource name in"=w817, "units"=w826, "set rate- string"=w821, "diameter(mm)-string"=w823, "address (string)"=w818) -> ("error out"=w827:errorcluster, "VISA resource name out"=w828:refnum<visa-resource-name>)  [unwired: 2 in]
              }
            }
          }
          frame 1 {
          }
          frame Default {
          }
          frame 3 {
          }
        }
        n341 = feedback #4(FALSE ("Motor Start/Stop")) -> (w626:bool)
        n342 = feedback-in #4("Pump1\nStart/Stop") -> ()
        n343 = Or(x="Pump1\nStart/Stop", y=w626) -> (x .or. y?=w625:bool)
        n344 = Build Array("Pump1\nStart/Stop", w626) -> (w640:bool[])
        n345 = Boolean Array To Number(Boolean array=w640) -> (number=w545:u32)
        n346 = call "Function_runNstop.vi"("VISA resource name in"=w591, "error in"=w592, "condition"=w545, "Server addr"=w593) -> ("VISA resource name out"=w587:refnum<visa-resource-name>, "error out"=w586:errorcluster)  [unwired: 6 in]
        n347 = Multiply(x="Target Vol1", y=0.001) -> (x*y=w619:dbl)
        n348 = Multiply(x="Target Vol2", y=0.001) -> (x*y=w570:dbl)
        n349 = Multiply(x="Target Vol3", y=0.001) -> (x*y=w563:dbl)
        n350 = feedback #5(FALSE ("Motor Start/Stop")) -> (w588:bool)
        n351 = feedback-in #5("Pump2\nStart/Stop") -> ()
        n352 = Build Array("Pump2\nStart/Stop", w588) -> (w590:bool[])
        n353 = Boolean Array To Number(Boolean array=w590) -> (number=w544:u32)
        n354 = Or(x="Pump2\nStart/Stop", y=w588) -> (x .or. y?=w576:bool)
        n355 = call "Function_runNstop.vi"("VISA resource name in"=w587, "error in"=w586, "condition"=w544, "Server addr"=w579) -> ("VISA resource name out"=w582:refnum<visa-resource-name>, "error out"=w539:errorcluster)  [unwired: 6 in]
        n356 = feedback #6(FALSE ("Motor Start/Stop")) -> (w583:bool)
        n357 = feedback-in #6("Pump3\nStart/Stop") -> ()
        n358 = Build Array("Pump3\nStart/Stop", w583) -> (w585:bool[])
        n359 = Boolean Array To Number(Boolean array=w585) -> (number=w543:u32)
        n360 = call "Function_runNstop.vi"("VISA resource name in"=w582, "error in"=w539, "condition"=w543, "Server addr"=w574) -> ("VISA resource name out"=w532:refnum<visa-resource-name>, "error out"=w533:errorcluster)  [unwired: 6 in]
        n361 = Or(x="Pump3\nStart/Stop", y=w583) -> (x .or. y?=w575:bool)
        n362 = case shown="True" w625 {
          tunnel: [w757 w760] -> w581
          tunnel: [w756 w759] -> w580
          tunnel: w532 -> [w757 w758]
          tunnel: w533 -> [w756 w762]
          tunnel: w593 -> [_ w763]
          tunnel: ["0" ("Vol Infused") w761] -> w624
          frame False {
          }
          frame True {
            n363 = property on="Direction1" class="CmbBox"() -> ("Value"=w764:string)  [unwired: 2 in, 2 out]
            n364 = call "Function_request_status.vi"("VISA resource name in"=w758, "error in"=w762, "Direction"=w764, "Server addr"=w763) -> ("Dispensed1"=w761:string, "VISA resource name out"=w760:refnum<visa-resource-name>, "error out"=w759:errorcluster)  [unwired: 5 in]
            "Dispensed1" <- w761
          }
        }
        n365 = Fract/Exp String To Number(string=w624) -> (number=w623:dbl)  [unwired: 3 in, 1 out]
        n366 = Subtract(x=w619, y=w623) -> (x-y=w622:dbl)
        n367 = Number To Fractional String(number=w622) -> (F-format string=w618:string)  [unwired: 3 in]
        n368 = Concatenate Strings(w618, "ML" ("string")) -> (→"Remains1":string)
        n369 = case shown="True" w576 {
          tunnel: [w685 w687] -> w578
          tunnel: [w684 w686] -> w577
          tunnel: w581 -> [w685 w690]
          tunnel: w580 -> [w684 w689]
          tunnel: w579 -> [_ w691]
          tunnel: ["0" ("Vol Infused") w688] -> w557
          frame False {
          }
          frame True {
            n370 = property on="Direction2" class="CmbBox"() -> ("Value"=w692:string)  [unwired: 2 in, 2 out]
            n371 = call "Function_request_status.vi"("VISA resource name in"=w690, "error in"=w689, "Direction"=w692, "Server addr"=w691) -> ("Dispensed1"=w688:string, "VISA resource name out"=w687:refnum<visa-resource-name>, "error out"=w686:errorcluster)  [unwired: 5 in]
            "Dispensed2" <- w688
          }
        }
        n372 = Fract/Exp String To Number(string=w557) -> (number=w573:dbl)  [unwired: 3 in, 1 out]
        n373 = Subtract(x=w570, y=w573) -> (x-y=w572:dbl)
        n374 = Number To Fractional String(number=w572) -> (F-format string=w569:string)  [unwired: 3 in]
        n375 = Concatenate Strings(w569, "ML" ("string")) -> (→"Remains2":string)
        n376 = case shown="True" w575 {
          tunnel: [w675 w677] -> w530
          tunnel: [w674 w676] -> w531
          tunnel: w578 -> [w675 w680]
          tunnel: w577 -> [w674 w679]
          tunnel: w574 -> [_ w681]
          tunnel: ["0" ("Vol Infused") w678] -> w556
          frame False {
          }
          frame True {
            n377 = property on="Direction3" class="CmbBox"() -> ("Value"=w682:string)  [unwired: 2 in, 2 out]
            n378 = call "Function_request_status.vi"("VISA resource name in"=w680, "error in"=w679, "Direction"=w682, "Server addr"=w681) -> ("Dispensed1"=w678:string, "VISA resource name out"=w677:refnum<visa-resource-name>, "error out"=w676:errorcluster)  [unwired: 5 in]
            "Dispensed3" <- w678
          }
        }
        n379 = Fract/Exp String To Number(string=w556) -> (number=w566:dbl)  [unwired: 3 in, 1 out]
        n380 = Subtract(x=w563, y=w566) -> (x-y=w565:dbl)
        n381 = Number To Fractional String(number=w565) -> (F-format string=w562:string)  [unwired: 3 in]
        n382 = Concatenate Strings(w562, "ML" ("string")) -> (→"Remains3":string)
        n383 = case shown="True" "Reset1" {
          tunnel: w531 -> [w665 w672]
          tunnel: w530 -> [w666 w671]
          tunnel: [w665 w668] -> w553
          tunnel: [w666 w667] -> w552
          frame False {
          }
          frame True {
            n384 = call "Function_reset.vi"("VISA resource name in"=w671, "error in"=w672, "Server addr"="3" ("trimmed string")) -> ("VISA resource name out"=w667:refnum<visa-resource-name>, "error out"=w668:errorcluster)  [unwired: 7 in]
            n385 = property on="Dispensed1" class="Str"("Value"="0" ("Vol Infused")) -> ()  [unwired: 2 in, 2 out]
          }
        }
        n386 = case shown="True" "Reset2" {
          tunnel: w553 -> [w657 w664]
          tunnel: w552 -> [w658 w663]
          tunnel: [w657 w660] -> w549
          tunnel: [w658 w659] -> w548
          frame False {
          }
          frame True {
            n387 = call "Function_reset.vi"("VISA resource name in"=w663, "error in"=w664, "Server addr"="1" ("trimmed string")) -> ("VISA resource name out"=w659:refnum<visa-resource-name>, "error out"=w660:errorcluster)  [unwired: 7 in]
            n388 = property on="Dispensed2" class="Str"("Value"="0" ("Vol Infused")) -> ()  [unwired: 2 in, 2 out]
          }
        }
        n389 = case shown="True" "Reset3" {
          tunnel: w549 -> [w650 w656]
          tunnel: w548 -> [w649 w651]
          tunnel: [w650 w653] -> w547
          tunnel: [w649 w652] -> w546
          frame False {
          }
          frame True {
            n390 = call "Function_reset.vi"("VISA resource name in"=w651, "error in"=w656, "Server addr"="2" ("trimmed string")) -> ("VISA resource name out"=w652:refnum<visa-resource-name>, "error out"=w653:errorcluster)  [unwired: 7 in]
            n391 = property on="Dispensed3" class="Str"("Value"="0" ("Vol Infused")) -> ()  [unwired: 2 in, 2 out]
          }
        }
        n392 = case shown="True" "Reset4" {
          tunnel: w547 -> [w642 w648]
          tunnel: w546 -> [w643 w647]
          tunnel: [w643 w645] -> w535
          tunnel: [w642 w644] -> w534
          frame False {
          }
          frame True {
            (unwired) "0" ("Vol Infused")
            n393 = call "Function_reset.vi"("VISA resource name in"=w647, "error in"=w648, "Server addr"="0" ("trimmed string")) -> ("VISA resource name out"=w645:refnum<visa-resource-name>, "error out"=w644:errorcluster)  [unwired: 7 in]
          }
        }
      }
      n394 = xnode "Close FPGA VI Reference"("FPGA VI Reference In"=w68, "error in"=w67) -> ()  [unwired: 1 out]
      n395 = VISA Close(VISA resource name=w47, error in (no error)=w51) -> (error out=w52:errorcluster)
      n396 = call <vilib>:"Simple Error Handler.vi"("error in (no error)"=w52) -> ()  [unwired: 4 in, 5 out]
      n397 = VISA Close(VISA resource name=w56, error in (no error)=w55) -> (error out=w57:errorcluster)
      n398 = call <vilib>:"Simple Error Handler.vi"("error in (no error)"=w57) -> ()  [unwired: 4 in, 5 out]
      "Baud Rate" <- w60
    }
    frame #2 {
      n399 = local read "Data File Ptr"() -> (w975:refnum<file>)
      n400 = Close File(refnum=w975) -> ()  [unwired: 1 in, 2 out]
    }
  }
